vi "FrontPanel.vi"() -> ()   [LabVIEW 2016]
doc: "This VI controls the blindpanel type GHS-2T-1T-700 for a CryoFree DR. Automatization control is embedded in the blindpanel. Keys can be manipulated from within this VI."
uses:
  <userlib>/LevyLab/Leiden Tools/Leiden to DSC/FP to DSC/Typedefs/FP-cluster.ctl
  <vilib>/Utility/file.llb/Write Delimited Spreadsheet (string).vi
  Lib/Lib.llb/ErrCodeStatusLkup.vi
  Lib/Lib.llb/Pfeiffer Vacuum.lvlib
panel:
  out "VIRef":T1 {"Array DataType" format="%.0x"; "WaveForm Type" format="%.0x"; "RefNum Type" format="%.0x"; "DataType" format="%.0x"}
  out "ControlNames":string[](array[string])
  in  "Toolbar":enum32{"Page 1", "Page 2"}(tab)
  in  "Load config":bool
  in  "Save config":bool
  in  "Start":bool
  in  "Stop":bool
  out "V":string
  out "PT2 Data":dbl[](array[numeric])
  in  "Restart PT on Error?":bool
  in  "Attempts":u16=6
  in  "Time delay":u16=60 format="%.0f s"
  out "Error Log":string[][](table)
  in  "Error panel":enum32{"Page 1"}(tab)
  out "PT2 error":errorcluster
  out "MG error":errorcluster
  out "PT1 error":errorcluster
  out "FP error":errorcluster
  out "PT1 Data":dbl[](array[numeric])
  in  "Main Panel":enum32{"Page 1", "Page 2"}(tab)
  out "PC":sgl
  out "P1":sgl format="%.1f"
  out "P2":sgl format="%.1f"
  out "P3":sgl format="%.1f"
  out "P4":sgl format="%.1f"
  out "P5":sgl format="%.1f"
  out "P6":sgl format="%.1f"
  out "P7":sgl format="%.1f"
  out "Flow":sgl format="%#_4f"
  out "P5 alarm":bool
  out "Pstill (P8)":dbl format="%.1e"
  in  "Main Panel":T2(tab)
  out "String 2":string
  out "String 4":string
  out "String":string
  out "String 3":string
  out "Mode":u16(ring) items=["AUTO MODE OFF", "START", "CONDENSING 3He", "CONDENSING 4He", "NORMAL CIRCULATION", "RECOVERY OF THE MIXTURE", "RECOVERY: BLOCKAGE OR OVERPRESSURE"]
  out "FLOW":sgl format="%#_3f"
  out "P5":sgl
  out "P4":sgl
  out "P3":sgl
  out "P1":sgl
  out "P2":sgl
  out "3He":sgl(slide) min=0 max=2 scale=0.0..2000.0 scale format="%.2f"
  out "4He":sgl(slide) min=0 max=2 scale=0.0..2000.0 scale format="%.2f"
  out "Panel ID":string
  in  "FP type":enum32{"OLD", "NEW"}(tab)
  in  "Buttons":T3
  out "LEDs":T4
  in  "Buttons 2":T3
  out "LEDs 2":T5
  out "PC":sgl caption="P COMP"
  in  "PT Start 2":bool
  in  "PT_stop 2":bool
  in  "PT2 Plots Select":T6
  out "PT2 Status":cluster{"Time":dbl[], "Value":dbl[]}[](graph)
  in  "PT_ResetValues 2":bool
  out "PT Error Code 2":i32 caption="PT Error Code"
  out "PT Error 2":string="NO ERROR" caption="PT Error"
  out "P High":cluster{dbl, dbl, dbl, dbl}(slide) scale=150.0..450.0
  out "P Low":cluster{dbl, dbl, dbl, dbl}(slide) scale=0.0..300.0
  out "P_avg 2":cluster{"Low":dbl, "High":dbl} caption="Average pressure"
  out "Helium":cluster{dbl, dbl, dbl, dbl}(slide) scale=0.0..95.0
  out "Water In":cluster{dbl, dbl, dbl, dbl}(slide) scale=0.0..35.0
  out "Water Out":cluster{dbl, dbl, dbl, dbl}(slide) scale=0.0..60.0
  out "PT Status":u16(ring) items=["Compressor OFF", "Compressor ON", ""]
  out "Motor":cluster{dbl, dbl}(slide) scale=0.0..30.0
  out "Oil":cluster{dbl, dbl, dbl, dbl}(slide) scale=0.0..60.0
  in  "PT1 Plots Select":T6
  out "PT1 Status 2":cluster{"Time":dbl[], "Value":dbl[]}[](graph)
  out "P Low":cluster{dbl, dbl, dbl, dbl}(slide) scale=0.0..300.0
  out "P High":cluster{dbl, dbl, dbl, dbl}(slide) scale=150.0..450.0
  out "P_avg":cluster{"Low":dbl, "High":dbl} caption="Average pressure"
  out "Motor":cluster{dbl, dbl}(slide) scale=0.0..30.0
  out "Oil":cluster{dbl, dbl, dbl, dbl}(slide) scale=0.0..60.0
  out "Helium":cluster{dbl, dbl, dbl, dbl}(slide) scale=0.0..95.0
  out "Water Out":cluster{dbl, dbl, dbl, dbl}(slide) scale=0.0..60.0
  out "Water In":cluster{dbl, dbl, dbl, dbl}(slide) scale=0.0..35.0
  out "PT Error Code":i32
  out "PT Error":string="NO ERROR"
  in  "PT_ResetValues":bool
  in  "PT Start":bool
  in  "PT_stop":bool
  out "PT Status":u16(ring) items=["Compressor OFF", "Compressor ON", ""]
  in  "MG Plots Select":T6
  in  "FP Plots Select":T6
  out "MaxiGauge":cluster{"Time":dbl[], "Value":dbl[]}[](graph)
  out "Front Panel":cluster{"Time":dbl[], "Value":dbl[]}[](graph)
  in  "Boolean 2":bool
  out "Maxigauge ID":string
  out "ForceSave":bool
  in  "Type":enum32{"Wet", "CF"}(radio)=enum."CF"
  in  "Button":u8
  out "SetControl":T7
  in  "S2":enum32{"Page 1"}(tab)
  in  "Reset Error 2":bool
  in  "S1":enum32{"Page 1"}(tab)
  in  "Reset Error":bool
  out "Cur Path":path
  in  "Side Panel":enum32{"Main", "Settings", "Advanced"}(tab)=enum."Settings"
  out "Sensors Status":T8={"String 8"="OK", "String 9"="OK", "String 10"="OK", "String 11"="OK", "String 12"="OK", "String 13"="OK"}
  in  "ADC scaling":T9={"P1"=2500.0, "P2"=2500.0, "P3"=2500.0, "P4"=2500.0, "P5"=2500.0, "P6"=2500.0, "P7"=2500.0, "Flow meter"=682.0, "PC"=10000.0} caption="Front panel ADC scaling factors" {"Flow meter" format="%#.4f"}
  in  "REC Settings":T10={"P6 low"=20, "P6 high"=1000, "P7 low"=20}
  in  "NCP5B Settings":cluster{"P6 low":u16}={"P6 low"=20}
  in  "NCP5 Settings":T10={"P6 low"=20, "P6 high"=1000, "P7 low"=20}
  in  "S1&2 Settings":cluster{"Enum":enum16{"OFF", "ON"}}
  in  "P5 Settings":cluster{"P6 low":u16, "P6 high":u16}={"P6 low"=20, "P6 high"=1000}
  out "REC limits":T11={"P5 warn"=20, "P5 rec"=20, "P5 res"=20}
  out "NCP5B limits":cluster{"P5 NC4":u16}={"P5 NC4"=20}
  out "NCP5 limits":T12={"P5 NC1"=20, "P5 NC2"=20, "P5 NC3"=20}
  out "S1&2 limits":cluster{"S1&S2":enum16{"OFF", "ON"}}
  out "P5 limits":cluster{"P5 C1":u16, "P5 C2":u16}={"P5 C1"=20, "P5 C2"=20}
  in  "P6&7 Settings":T13={"P6 low"=20, "P6 high"=1600, "P7 low"=20, "P7 high"=1610}
  out "P6&7 limits":T13={"P6 low"=20, "P6 high"=20, "P7 low"=20, "P7 high"=20}
  in  "SET VALUES":bool
  out "MG pressures":T14 {"Channel 1" format="%-7.2e mbar"; "Channel 1" format="%-7.2e mbar"; "Channel 1" format="%-7.2e mbar"; "Channel 1" format="%-7.2e mbar"; "Channel 1" format="%-7.2e mbar"; "Channel 1" format="%-7.2e mbar"}
  out "Cluster":T15={"String 2"="\"\"", "String 3"="", "String 4"="", "String 5"="", "String 6"="", "String 7"=""}
  in  "Log Options":T16={"Plot data "=TRUE, "Every1"=1.0, "Save to log"=TRUE, "Every  2"=1.0, "AVS_Path 2"=path "C:/avs-47", "AVS_FName"="logFP", "Filename suffix"="_%Y-%m-%d-%H-%M-%S", "NewFevery"=7, "Time Units"=enum."Days", "Date Format"="%Y-%m-%d %H:%M:%S", "Averages"=4} caption="Data Logging \nOptions" {"Every  2" format="%#_g min"; "Every1" format="%#_g min"}
  in  "Configuration":T17={"FP port"="COM3", "MG port"="COM4", "PT1 Enabled?"=FALSE, "MG  channel P8"=65535, "Stop auto recovery if still is empty"=FALSE, "PT1 port"="COM2", "MG Enabled?"=TRUE, "PT1 Address"=16, "S1 Enabled?"=FALSE, "S1 port"="COM2", "S2 Enabled?"=FALSE, "S2 port"="COM2", "Device address S1"=1, "Device address S2"=2, "PT1 Bauds"=115200, "PT2 Enabled?"=FALSE, "PT2 port"="COM2", "PT2 Address"=16, "PT2 Bauds"=115200, "FP baud rate"=9600} {"PT2 Address" min=16 max=126 step=1; "MG  channel P8" items=["Channel 1", "Channel 2", "Channel 3", "Channel 4", "Channel 5", "Channel 6"]; "PT1 Address" min=16 max=126 step=1}
  in  "SendCMD":bool caption="Send"
  out "Response":string
  in  "Command":string
  out "SP reached? 2":bool
  in  "Cond1":bool
  in  "Delay Time":u32=30 caption="For a time delay of" format="%.0f min"
  in  "MG  channel":u16(ring)=65535 caption="MaxiGauge" items=["Channel 1", "Channel 2", "Channel 3", "Channel 4", "Channel 5", "Channel 6"]
  out "SP reached? 3":bool
  in  "P threshold":dbl=0.0005 caption="<" format="%#_2g mbar"
  in  "Cond2":bool
  out "SP reached?":bool
  out "Delay Timer":u32=10 caption="Timer" format="%<%M:%S>t"
  in  "EnableAutoCond":bool caption="Start"
  in  "Autoconf":bool caption="Autoconfigure"
  out "MG Data":dbl[](array[numeric]) format="%.3e"
  out "FP Data":sgl[](array[numeric]) format="%.2f"
  out "FP Status bits":u32[](array[numeric])
  out "Attempts Counter":u16
  # "Error log"
  # "Front panel status"
  # "MaxiGauge status"
  # "Pulse Tube 1 status"
  # "Pulse Tube 2 status"
  # "Leiden Cryogenics"
  # "to \nair"
  # "N.C."
  # "from\novc"
  # "from\nivc"
  # "from still"
  # "to 3He\nin-1"
  # "to 3He\nin-2"
  # "P8"
  # "AUX 1"
  # "MIXTURE\nCOMPRESSOR"
  # "M2"
  # "P6"
  # "M3"
  # "M1"
  # "AUX PORT-1"
  # "P7"
  # "TRAP"
  # "AUX TRAP"
  # "To \nAir"
  # "From\nIVC"
  # "From Still"
  # "To 3He\nin-1"
  # "To 3He\nin-2"
  # "To \nAir"
  # "N.C."
  # "from\novc"
  # "from\nivc"
  # "from still"
  # "to 3He\nin-1"
  # "to 3He\nin-2"
  # "Leiden Cryogenics"
  # "to \nair"
  # "N.C."
  # "from\novc"
  # "from\nivc"
  # "from still"
  # "to 3He\nin-1"
  # "to 3He\nin-2"
  # "P8"
  # "M2"
  # "P6"
  # "M3"
  # "TRAP"
  # "AUX TRAP"
  # "M1"
  # "AUX PORT-1"
  # "P7"
  # "AUX 1"
  # "To \nAir"
  # "From\nIVC"
  # "From Still"
  # "To 3He\nin-1"
  # "to 3He\nin-1"
  # "To 3He\nin-2"
  # "to \nair"
  # "N.C."
  # "from\novc"
  # "from\nivc"
  # "from still"
  # "to 3He\nin-2"
  # "Pulse Tube 1"
  # "Pulse Tube 2"
  # "Front Panel"
  # "MaxiGauge"
  # "Turbo2 (S2)"
  # "Turbo1 (S1)"
  # "MaxiGauge"
  # "#"
  # "NAME"
  # "PRESSURE"
  # "STATUS"
  # "1"
  # "2"
  # "3"
  # "4"
  # "5"
  # "6"
  # "Automatic mode pressure limits"
  # "Warning: These values influence the operation of the GHS in automatic mode. Please refer to the operation manual and consult with Leiden Cryogenics before changing them."
  # "NAME"
  # "FW"
  # "NEW"
  # "DESCRIPTION"
  # "Stop condensing 4He"
  # "Stop recovering 4He"
  # "Stop condensing 3He"
  # "Stop recovering 3He"
  # "Condensing->open 12"
  # "Condensing->close 9/12"
  # "Condensing->run S1&S2"
  # "NC->open second line"
  # "NC->start MC"
  # "NC->open aux. trap"
  # "NC->stop MC, close 7"
  # "All->P5 alarm"
  # "All->switch to recovery"
  # "All->reset"
  # "Front panel ADC scaling factors"
  # "Data Logging and Plotting"
  # "Front Panel"
  # "MaxiGauge"
  # "Pulse Tube 1"
  # "Pulse Tube 2"
  # "Turbo 1 (S1) (Pfeiffer HiPACE only)"
  # "Turbo2 (S2) (Pfeiffer HiPACE only)"
  # "Automatic condensing"
  # "Start condensing when"
  # "and wait"
  # "Send command to Front Panel"
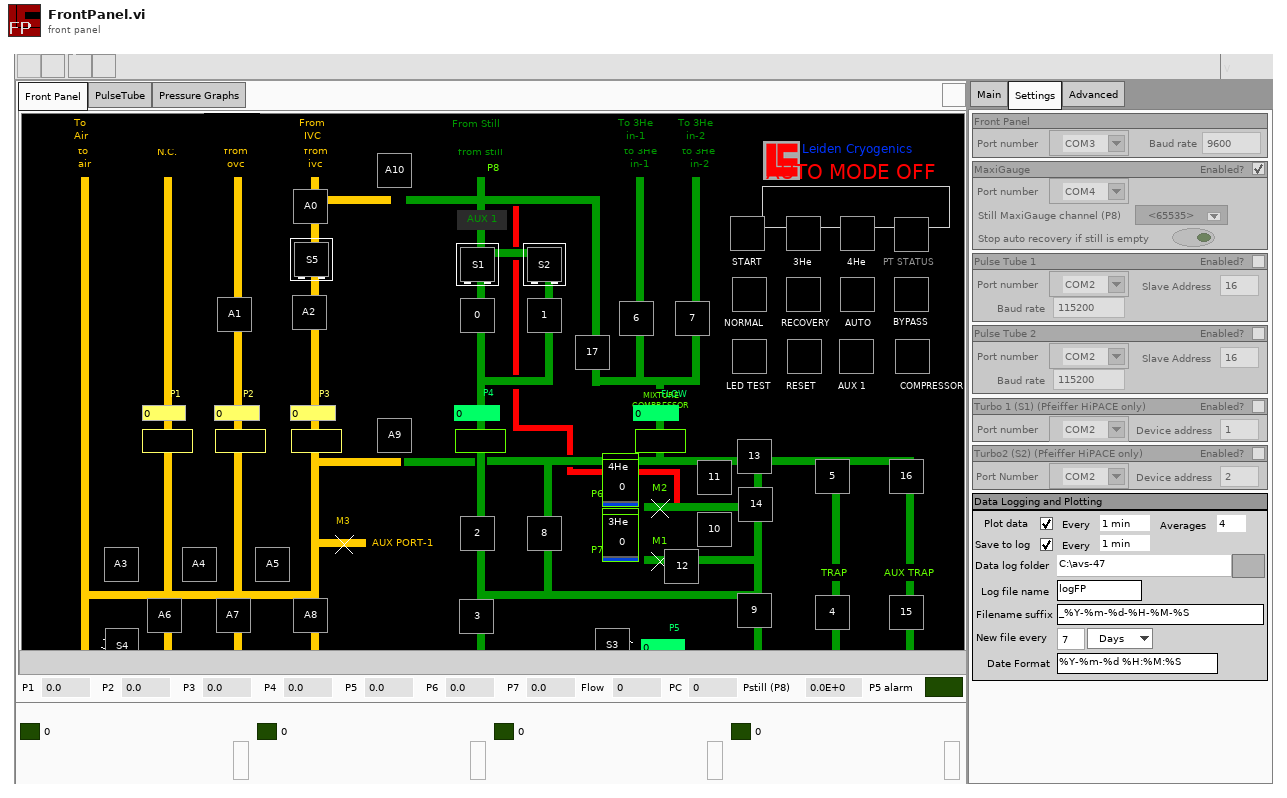
[diagram p1: front panel]
types:
  T1 = cluster{"Control Ref ID":refnum<vi>[], "Full Name":string[], "ClassID":enum16{"<Null>", "1", "2", "Generic", "Decoration", "Text", "Control", "ColorBox", "Boolean", "RefNum", "Variant", "Path", "ListBox", "Table", "Array", "Picture", "ActiveXContainer", "Numeric", "Digital", "NamedNumeric", "ColorRamp", "Slide", "GraphOrChart", "WaveformChart", "WaveformGraph", "IntensityChart", "IntensityGraph", "String", "IOName", "ComboBox", "Cluster", "Panel", "Knob", "NumWithScale", "Ring", "Enum", "GObject", "Plot", "Cursor", "NumericText", "Scale", "ColorScale", "GraphScale", "ColorGraphScale", "TypedRefNum", "OldKnobScale", "MCListbox", "MeasureData", "BVTag", "DAQName", "VISAName", "IVIName", "SlideScale", "TabControl", "Page", "TabArrayTabControl", "ConPane", "57", "58", "59", "60", "61", "62", "63", "64", "SubPanel", "TreeControl", "67", "68", "69", "70", "71", "72", "73", "74", "75", "SplitterBar"}[], "Short Name":string[], "DataType":enum8{"<Null>", "I8", "I16", "I32", "I64", "U8", "U16", "U32", "U64", "SGL", "DBL", "EXT", "CSG", "CDB", "CXT", "0x0F", "0x10", "0x11", "0x12", "0x13", "0x14", "Enum U8", "Enum U16", "Enum U32", "Enum U64", "SGL PQ", "DBL PQ", "EXT PQ", "CSG PQ", "CDB PQ", "CXT PQ", "0x1F", "0x20", "Boolean", "0x22", "0x23", "0x24", "0x25", "0x26", "0x27", "0x28", "0x29", "0x2A", "0x2B", "0x2C", "0x2D", "0x2E", "0x2F", "String", "0x31", "Path", "Pict", "0x34", "0x35", "0x36", "DAQ", "0x38", "0x39", "0x3A", "0x3B", "0x3C", "0x3D", "0x3E", "0x3F", "Array", "0x41", "0x42", "0x43", "0x44", "0x45", "0x46", "0x47", "0x48", "0x49", "0x4A", "0x4B", "0x4C", "0x4D", "0x4E", "0x4F", "Cluster", "0x51", "0x52", "Variant", "Waveform", "0x55", "0x56", "0x57", "0x58", "0x59", "0x5A", "0x5B", "0x5C", "0x5D", "0x5E", "0x5F", "0x60", "0x61", "0x62", "0x63", "0x64", "0x65", "0x66", "0x67", "0x68", "0x69", "0x6A", "0x6B", "0x6C", "0x6D", "0x6E", "0x6F", "Refnum"}[], "RefNum Type":enum8{"Generic", "Datalog File Refnum", "Byte Stream File Refnum", "Device Refnum", "Occurence Refnum", "TCP Connection Refnum", "VISA Refnum (Obsolete)", "Automation Renum", "VI Server Refnum", "Menu Refnum", "IVI Refnum (Obsolete)", "IMAQ Session", "0x0C", "Datasocket Refnum", "VISA Resource", "IVI Logical Name", "UDP Connection Refnum", "Notifier Refnum", "Queue Refnum", "IrDA Refnum", "Hardware Plugin Refnum", "Hardware Plugin Tag Refnum", "DAQmx Refnum", "Event Registration Refnum", ".NET Refnum", "User Event Refnum", "0x1A", "Event Callback", "0x1C", "0x1D", "Only Used Internal to LabVIEW", "Bluetooth", "Data Value References", "RT FIFO", "TDM Streaming"}[], "WaveForm Type":enum8{"<Not a Waveform Type>", "0x01", "Analog 16-bit signed", "Analog Double-Precision", "0x04", "Analog Single Precision", "Timestamp", "Digital Data", "Digital Waveform", "Dynamic Data", "Analog Extended-Precision", "Analog 8-bit unsigned", "Analog 16-bit unsigned", "Analog 32-bit unsigned", "Analog 8-bit signed", "Analog 32-bit signed", "Analog Complex Single-Precision", "Analog Complex Double-Precision", "Analog Complex Extended Precision", "Analog 64-bit signed", "Analog 64-bit unsigned"}[], "Parent":i32[], "Array DataType":enum8{"<Null>", "I8", "I16", "I32", "I64", "U8", "U16", "U32", "U64", "SGL", "DBL", "EXT", "CSG", "CDB", "CXT", "0x0F", "0x10", "0x11", "0x12", "0x13", "0x14", "Enum U8", "Enum U16", "Enum U32", "Enum U64", "SGL PQ", "DBL PQ", "EXT PQ", "CSG PQ", "CDB PQ", "CXT PQ", "0x1F", "0x20", "Boolean", "0x22", "0x23", "0x24", "0x25", "0x26", "0x27", "0x28", "0x29", "0x2A", "0x2B", "0x2C", "0x2D", "0x2E", "0x2F", "String", "0x31", "Path", "Pict", "0x34", "0x35", "0x36", "DAQ", "0x38", "0x39", "0x3A", "0x3B", "0x3C", "0x3D", "0x3E", "0x3F", "Array", "0x41", "0x42", "0x43", "0x44", "0x45", "0x46", "0x47", "0x48", "0x49", "0x4A", "0x4B", "0x4C", "0x4D", "0x4E", "0x4F", "Cluster", "0x51", "0x52", "Variant", "Waveform", "0x55", "0x56", "0x57", "0x58", "0x59", "0x5A", "0x5B", "0x5C", "0x5D", "0x5E", "0x5F", "0x60", "0x61", "0x62", "0x63", "0x64", "0x65", "0x66", "0x67", "0x68", "0x69", "0x6A", "0x6B", "0x6C", "0x6D", "0x6E", "0x6F", "Refnum"}[], "Owning VI":refnum<vi>[], "Active?":bool[]}
  T2 = enum32{"Front Panel", "PulseTube", "Pressure Graphs"}
  T3 = cluster{"baux2":bool, "bBypass":bool, "b15":bool, "b16":bool, "NC 0":bool, "baux1":bool, "b4":bool, "NC 1":bool, "b5":bool, "breset":bool, "NC 2":bool, "b9":bool, "b14":bool, "NC 3":bool, "b13":bool, "bledtest":bool, "NC 4":bool, "b12":bool, "b10":bool, "NC 5":bool, "b11":bool, "bA0":bool, "NC 9":bool, "b7":bool, "bS3":bool, "NC 12":bool, "b6":bool, "b17":bool, "NC 13":bool, "b8":bool, "b1":bool, "NC 14":bool, "bS2":bool, "b3":bool, "NC 15":bool, "b2":bool, "b0":bool, "NC 16":bool, "bS1":bool, "bA9":bool, "NC 17":bool, "bA8":bool, "bA2":bool, "NC 6":bool, "bs5":bool, "bA10":bool, "NC 7":bool, "bstart":bool, "bA5":bool, "NC 8":bool, "bA7":bool, "bA1":bool, "NC 10":bool, "bauto":bool, "bA4":bool, "NC 11":bool, "bA6":bool, "bS4":bool, "NC 18":bool, "bA3":bool, "b3he":bool, "b4he":bool, "bnorm":bool, "brecov":bool}
  T4 = cluster{"COMPR/AUX 2":bool, "BYPASS":bool, "15":bool, "16":bool, "NC 0":bool, "AUX 1":bool, "4":bool, "NC 1":bool, "5":bool, "RESET":bool, "NC 2":bool, "9":bool, "14":bool, "NC 3":bool, "13":bool, "LED TEST":bool, "NC 4":bool, "12":bool, "10":bool, "NC 5":bool, "11":bool, "A0":bool, "NC 12":bool, "7":bool, "S3":bool, "NC 13":bool, "6":bool, "17":bool, "NC 14":bool, "8":bool, "1":bool, "NC 15":bool, "S2":bool, "3":bool, "NC 16":bool, "2":bool, "0":bool, "NC 17":bool, "S1":bool, "A9":bool, "NC 6":bool, "A8":bool, "A2":bool, "NC 7":bool, "S5":bool, "A10":bool, "NC 8":bool, "START":bool, "A5":bool, "NC 9":bool, "A7":bool, "A1":bool, "NC 10":bool, "AUTO":bool, "A4":bool, "NC 11":bool, "A6":bool, "S4":bool, "NC 18":bool, "A3":bool, "3He":bool, "4He":bool, "NORMAL":bool, "RECOVERY":bool, "PT STATUS":bool}
  T5 = cluster{"COMPR/AUX 2":bool, "BYPASS":bool, "15":bool, "16":bool, "AUX 1":bool, "AUX 1":bool, "4":bool, "AUX 2":bool, "5":bool, "RESET":bool, "AUX 3":bool, "9":bool, "14":bool, "NC 3":bool, "13":bool, "LED TEST":bool, "NC 4":bool, "12":bool, "10":bool, "NC 5":bool, "11":bool, "A0":bool, "NC 12":bool, "7":bool, "S3":bool, "NC 13":bool, "6":bool, "17":bool, "NC 14":bool, "8":bool, "1":bool, "NC 15":bool, "S2":bool, "3":bool, "NC 16":bool, "2":bool, "0":bool, "NC 17":bool, "S1":bool, "A9":bool, "NC 6":bool, "A8":bool, "A2":bool, "NC 7":bool, "S5":bool, "A10":bool, "NC 8":bool, "START":bool, "A5":bool, "NC 9":bool, "A7":bool, "A1":bool, "NC 10":bool, "AUTO":bool, "A4":bool, "NC 11":bool, "A6":bool, "S4":bool, "NC 18":bool, "A3":bool, "3He":bool, "4He":bool, "NORMAL":bool, "RECOVERY":bool, "PT STATUS":bool}
  T6 = cluster{"Boolean":bool, "Boolean 2":bool, "Boolean 3":bool, "Boolean 4":bool, "Boolean 5":bool, "Boolean 6":bool, "Boolean 7":bool, "Boolean 8":bool}
  T7 = cluster{"Name":string, "Scalar":string, "Array":string[][]}
  T8 = cluster{"String 8":string, "String 9":string, "String 10":string, "String 11":string, "String 12":string, "String 13":string}
  T9 = cluster{"P1":dbl, "P2":dbl, "P3":dbl, "P4":dbl, "P5":dbl, "P6":dbl, "P7":dbl, "Flow meter":dbl, "PC":dbl}
  T10 = cluster{"P6 low":u16, "P6 high":u16, "P7 low":u16}
  T11 = cluster{"P5 warn":u16, "P5 rec":u16, "P5 res":u16}
  T12 = cluster{"P5 NC1":u16, "P5 NC2":u16, "P5 NC3":u16}
  T13 = cluster{"P6 low":u16, "P6 high":u16, "P7 low":u16, "P7 high":u16}
  T14 = cluster{"Channel 1":dbl, "Channel 1":dbl, "Channel 1":dbl, "Channel 1":dbl, "Channel 1":dbl, "Channel 1":dbl}
  T15 = cluster{"String 2":string, "String 3":string, "String 4":string, "String 5":string, "String 6":string, "String 7":string}
  T16 = cluster{"Plot data ":bool, "Every1":dbl, "Save to log":bool, "Every  2":dbl, "AVS_Path 2":path, "AVS_FName":string, "Filename suffix":string, "NewFevery":u32, "Time Units":enum16{"Minutes", "Hours", "Days"}, "Date Format":string, "Averages":i32}
  T17 = cluster{"FP port":refnum<visa-resource-name>, "MG port":refnum<visa-resource-name>, "PT1 Enabled?":bool, "MG  channel P8":u16, "Stop auto recovery if still is empty":bool, "PT1 port":refnum<visa-resource-name>, "MG Enabled?":bool, "PT1 Address":u8, "S1 Enabled?":bool, "S1 port":refnum<visa-resource-name>, "S2 Enabled?":bool, "S2 port":refnum<visa-resource-name>, "Device address S1":u8, "Device address S2":u8, "PT1 Bauds":u32, "PT2 Enabled?":bool, "PT2 port":refnum<visa-resource-name>, "PT2 Address":u8, "PT2 Bauds":u32, "FP baud rate":u32}
  T18 = typedef "FP-cluster.ctl" = cluster{"FP Data":sgl[], "MG Data":dbl[], "PT Data":dbl[], "FP Status Bits":u32[], "Mode":u16}
  T19 = cluster{"error":bool, "code":i32, "source":string}
  T20 = cluster{"FP Data[0]":sgl, "FP Data[1]":sgl, "FP Data[2]":sgl, "FP Data[3]":sgl, "FP Data[4]":sgl, "FP Data[5]":sgl, "FP Data[6]":sgl, "FP Data[7]":sgl, "FP Data[8]":sgl}
  T21 = enum32{"Page Enabled", "Page Disabled", "Page Disabled & Grayed"}
  T22 = enum32{"invalid app kind", "Development System", "Run Time System", "Student Edition", "Embedded LabVIEW", "Evaluation", "Custom"}
  T23 = enum32{"HKEY_CLASSES_ROOT", "HKEY_CURRENT_USER", "HKEY_LOCAL_MACHINE", "HKEY_USERS", "HKEY_PERFORMANCE_DATA", "HKEY_CURRENT_CONFIG", "HKEY_DYN_DATA"}
  T24 = cluster{"Array[0]":string, "Array[1]":string, "Array[2]":string, "Array[3]":string, "Array[4]":string, "Array[5]":string}
  T25 = cluster{"array of 4 x 16 bit unsigned[0]":u16, "array of 4 x 16 bit unsigned[1]":u16, "array of 4 x 16 bit unsigned[2]":u16, "array of 4 x 16 bit unsigned[3]":u16}
  T26 = cluster{"array of 2 x 16 bit unsigned[0]":u16, "array of 2 x 16 bit unsigned[1]":u16}
  T27 = cluster{"array of 3 x 16 bit unsigned[0]":u16, "array of 3 x 16 bit unsigned[1]":u16, "array of 3 x 16 bit unsigned[2]":u16}
  T28 = typedef "LVRectTypeDef.ctl" = cluster{"Left":i16, "Top":i16, "Right":i16, "Bottom":i16}
  T29 = cluster{"[0]":bool, "[1]":bool, "[2]":bool, "[3]":bool, "[4]":bool, "[5]":bool, "[6]":bool, "[7]":bool, "[8]":bool, "[9]":bool, "[10]":bool, "[11]":bool, "[12]":bool, "[13]":bool, "[14]":bool, "[15]":bool, "[16]":bool, "[17]":bool, "[18]":bool, "[19]":bool, "[20]":bool, "[21]":bool, "[22]":bool, "[23]":bool, "[24]":bool, "[25]":bool, "[26]":bool, "[27]":bool, "[28]":bool, "[29]":bool, "[30]":bool, "[31]":bool, "[32]":bool, "[33]":bool, "[34]":bool, "[35]":bool, "[36]":bool, "[37]":bool, "[38]":bool, "[39]":bool, "[40]":bool, "[41]":bool, "[42]":bool, "[43]":bool, "[44]":bool, "[45]":bool, "[46]":bool, "[47]":bool, "[48]":bool, "[49]":bool, "[50]":bool, "[51]":bool, "[52]":bool, "[53]":bool, "[54]":bool, "[55]":bool, "[56]":bool, "[57]":bool, "[58]":bool, "[59]":bool, "[60]":bool, "[61]":bool, "[62]":bool, "[63]":bool, "[64]":bool}
  T30 = cluster{"Dict. Var":u16, "Description":string, "Values":i32[]}[]
  T31 = cluster{"[3]":dbl, "[3]":dbl, "[3]":dbl, "Values[3] 2":dbl}
  T32 = cluster{"[1]":dbl, "[1]":dbl, "[1]":dbl, "Values[1] 2":dbl}
  T33 = cluster{"Values[0]":dbl, "Values[0]":dbl, "Values[0]":dbl, "Values[0] 2":dbl}
  T34 = cluster{"error":bool, "code":i32, "error source":string}
  T35 = cluster{"sensor status info[0]":string, "sensor status info[1]":string, "sensor status info[2]":string, "sensor status info[3]":string, "sensor status info[4]":string, "sensor status info[5]":string}
  T36 = cluster{"Filterred[0]":dbl, "Filterred[1]":dbl, "Filterred[2]":dbl, "Filterred[3]":dbl, "Filterred[4]":dbl, "Filterred[5]":dbl}
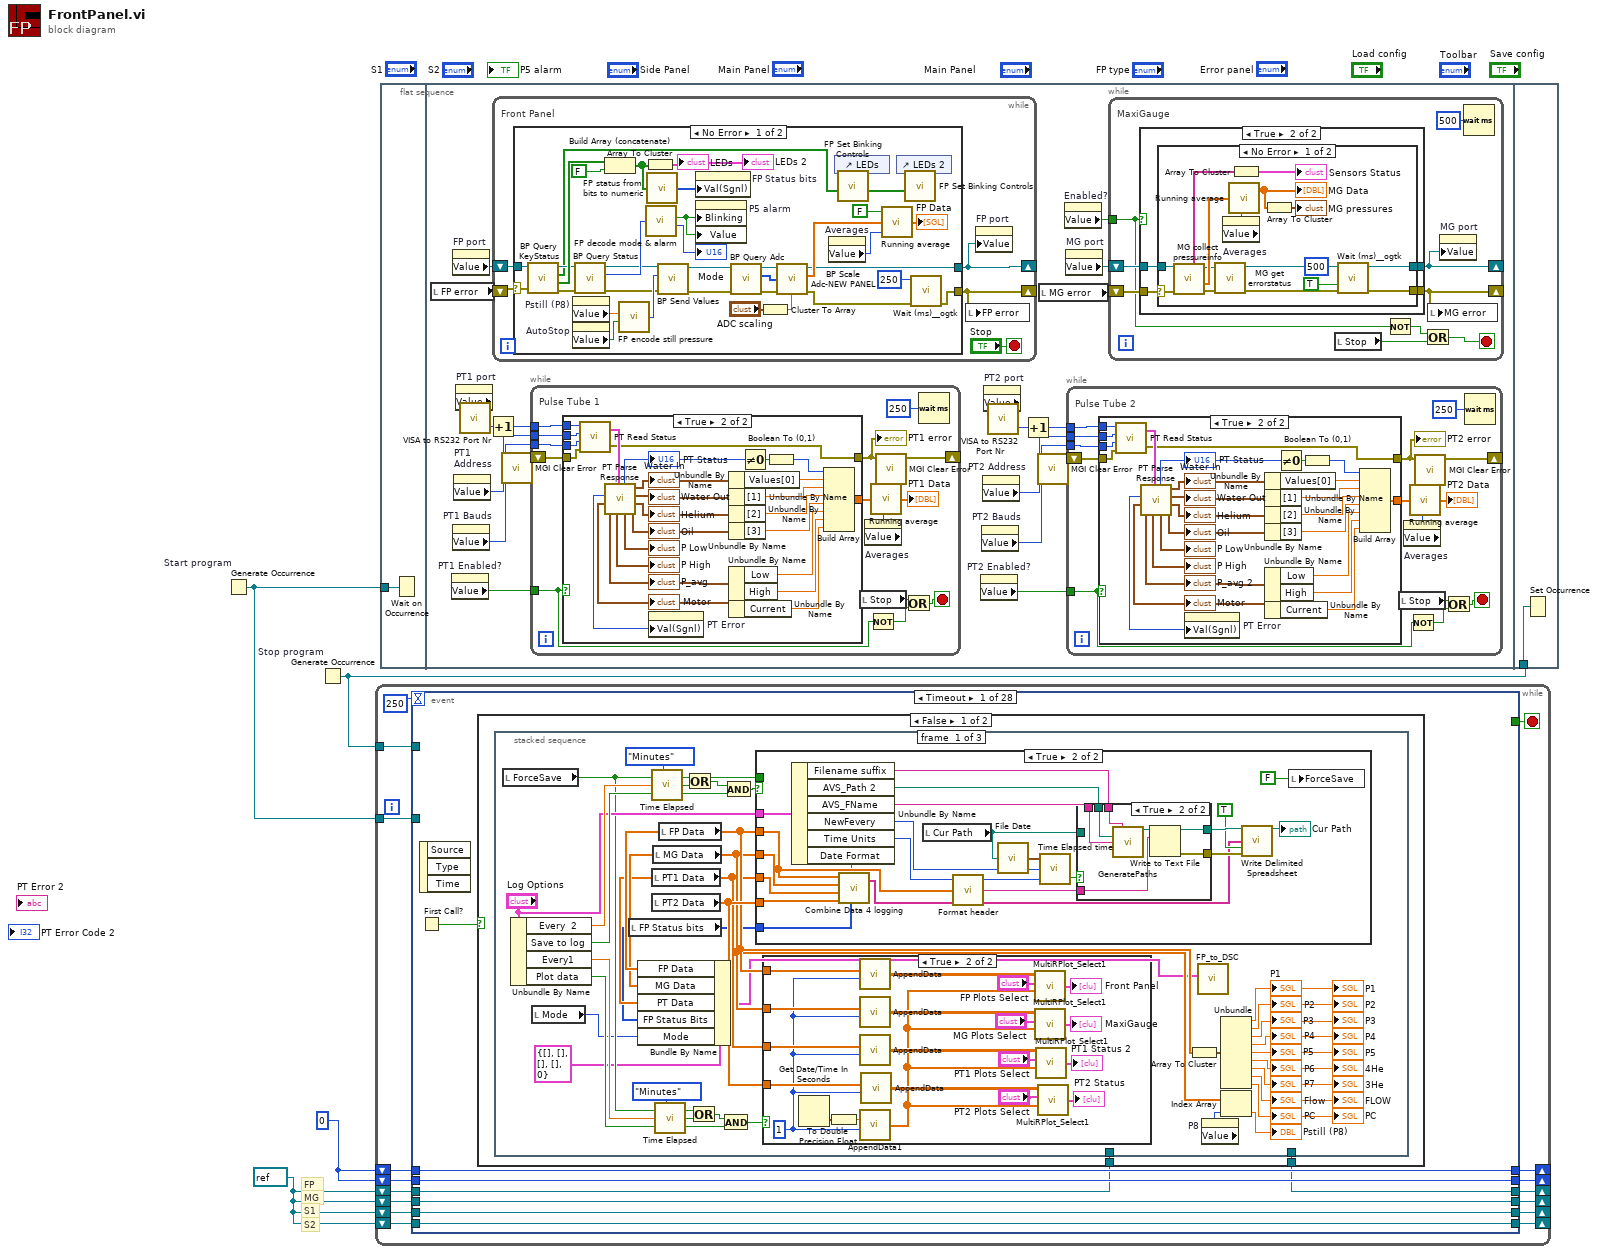
[diagram p0: block diagram]
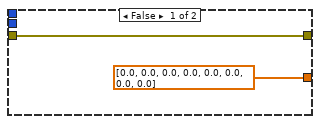
[diagram p2: hidden frame]
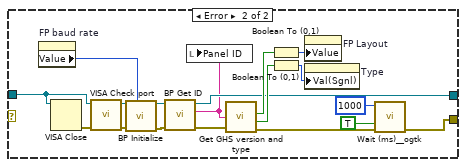
[diagram p3: hidden frame]
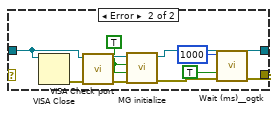
[diagram p5: hidden frame]
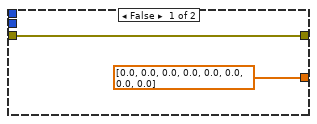
[diagram p6: hidden frame]
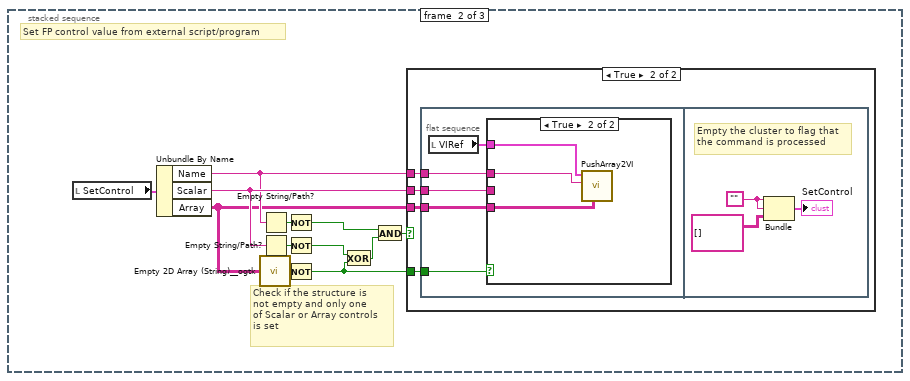
[diagram p10: hidden frame]
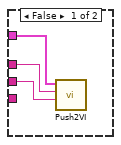
[diagram p12: hidden frame]
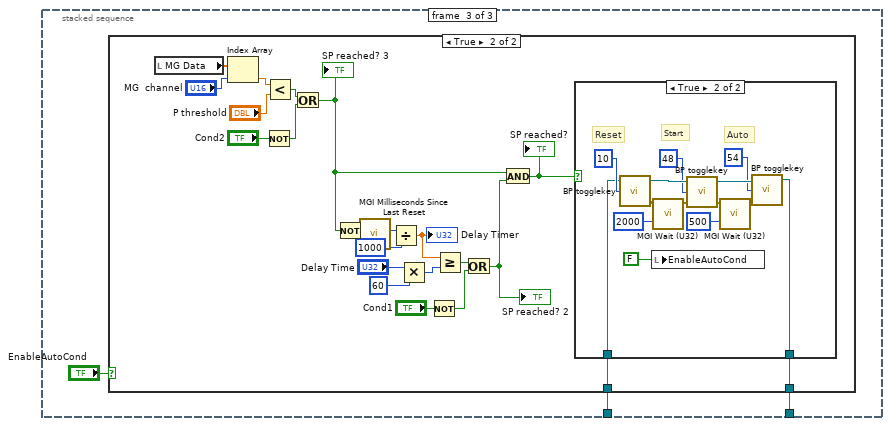
[diagram p13: hidden frame]
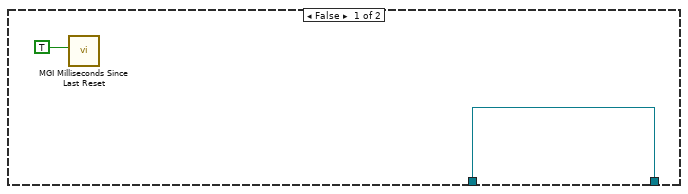
[diagram p14: hidden frame]
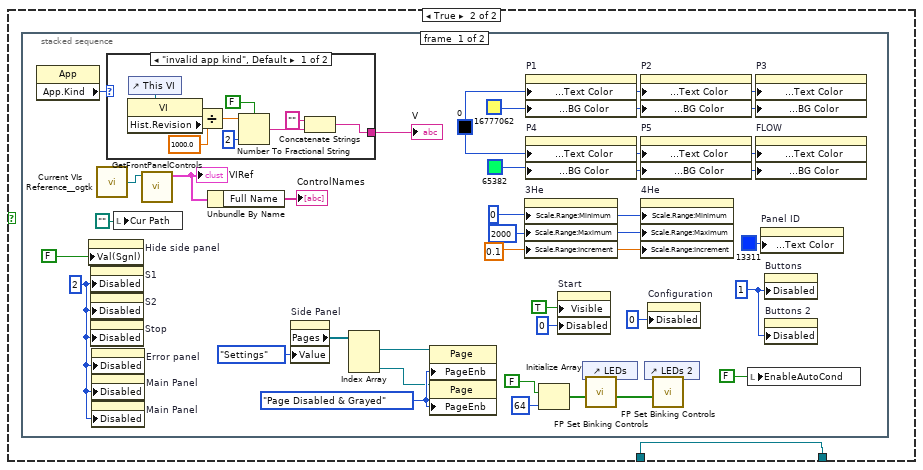
[diagram p16: hidden frame]
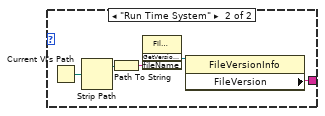
[diagram p17: hidden frame]
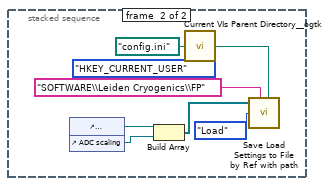
[diagram p18: hidden frame]
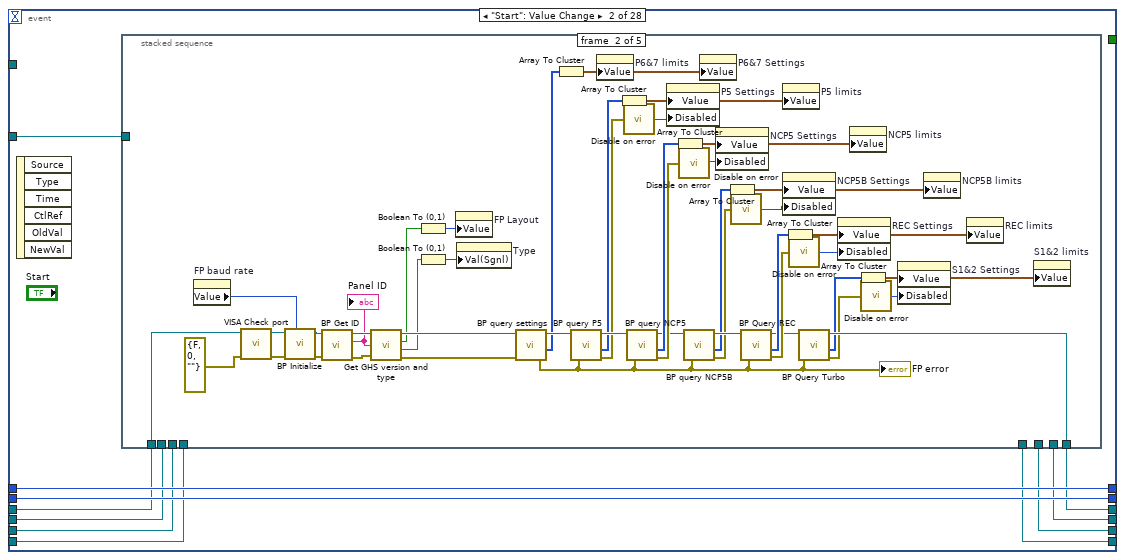
[diagram p19: hidden frame]
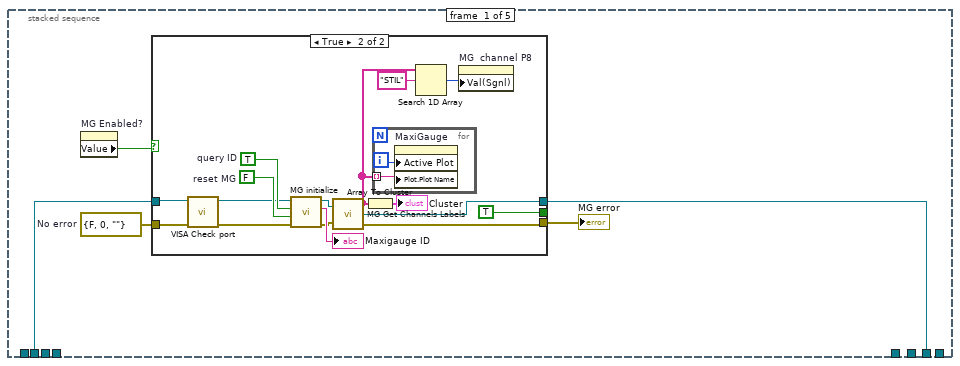
[diagram p20: hidden frame]
diagram:
  w3 = refnum<visa-resource-name> refnum ("PT port")
  w1 = u8 0
  # "S2"
  # "S1"
  # "FP"
  # "MG"
  n1 = Generate Occurrence "Start program"() -> (w4:refnum<k4>)
  n2 = Generate Occurrence "Stop program"() -> (w2:refnum<k4>)
  n3 = while {
    shift-right: [w12] -> _
    shift-left: w3 -> [w18]
    shift-right: [w16] -> _
    shift-left: w3 -> [w17]
    tunnel: w4 -> [w15]
    shift-right: [w13] -> _
    shift-left: w1 -> [w14]
    shift-right: [w9] -> _
    shift-left: w3 -> [w11]
    shift-right: [w8] -> _
    shift-left: w3 -> [w10]
    tunnel: w2 -> [w7]
    shift-right: [w5] -> _
    shift-left: w1 -> [w6]
    stop <- w20 stop-if-true
    n4 = event shown="[0] Timeout" {
      selector: _ -> [_ _ _ _ _ _ _ _ _ _ _ _ _ _ _ _ _ _ _ _ _ _ _ _ _ _ _ _]
      dyn-events: _ -> [_ _ _ _ _ _ _ _ _ _ _ _ _ _ _ _ _ _ _ _ _ _ _ _ _ _ _ _]
      timeout: 250 -> [_ _ _ _ _ _ _ _ _ _ _ _ _ _ _ _ _ _ _ _ _ _ _ _ _ _ _ _]
      tunnel: [_ _ TRUE _ _ _ _ _ _ _ _ _ _ _ _ _ _ _ _ _ _ _ _ _ _ _ _ _] -> w20
      tunnel: w18 -> [w22 w244 w349 w373 w382 w391 w400 w412 w443 w452 w458 w471 w485 w489 w582 w591 w601 w620 w634 w654 w664 w679 w686 w694 w702 w713 w725 w746]
      tunnel: w17 -> [w24 w246 w348 w372 w381 w390 w399 w411 w442 w451 w456 w469 w483 w493 w581 w590 w602 w619 w633 w653 w663 w678 w687 w695 w701 w712 w723 w749]
      tunnel: [w24 w245 w343 w372 w381 w390 w399 w411 w442 w451 w456 w469 w483 w493 w581 w590 w600 w619 w633 w653 w663 w678 w687 w695 w701 w712 w723 w749] -> w16
      tunnel: w15 -> [_ w242 _ _ _ _ _ _ _ _ _ _ _ _ _ _ _ _ _ _ _ _ _ _ _ _ _ _]
      tunnel: w14 -> [w27 w247 _ w371 w380 w389 w398 w408 w441 w450 w464 w476 w487 w492 w580 w592 _ w621 w635 w652 w665 w675 w685 w693 w703 w714 w724 w751]
      tunnel: [w27 w247 w344 w371 w380 w389 w398 w408 w441 w450 w464 w476 w487 w492 w580 w592 w603 w621 w635 w652 w665 w675 w685 w693 w703 w714 w724 w751] -> w13
      tunnel: [w21 w243 w343 w373 w382 w391 w400 w412 w443 w452 w457 w470 w484 w488 w582 w591 w606 w620 w634 w654 w664 w679 w686 w694 w702 w713 w725 w745] -> w12
      tunnel: w11 -> [w26 w241 w347 w370 w379 w388 w397 w404 w440 w449 w455 w468 w482 w491 w579 w589 w599 w618 w632 w651 w662 w677 w689 w696 w700 w711 w722 w748]
      tunnel: w10 -> [w25 w240 w346 w369 w378 w387 w396 w403 w439 w448 w454 w467 w481 w490 w578 w588 w597 w617 w631 w650 w661 w676 w688 w697 w699 w710 w721 w747]
      tunnel: [w26 w239 w343 w370 w379 w388 w397 w404 w440 w449 w455 w468 w482 w491 w579 w589 w598 w618 w632 w651 w662 w677 w683 w696 w700 w711 w722 w748] -> w9
      tunnel: [w25 w238 w343 w369 w378 w387 w396 w403 w439 w448 w454 w467 w481 w490 w578 w588 w596 w617 w631 w650 w661 w676 w688 w691 w699 w710 w721 w747] -> w8
      tunnel: w7 -> [_ _ w345 _ _ _ _ _ _ _ _ _ _ _ _ _ _ _ _ _ _ _ _ _ _ _ _ _]
      tunnel: w6 -> [w23 w248 _ w368 w377 w386 w395 w402 w438 w447 w463 w477 w486 w495 w577 w587 _ w608 w630 w640 w657 w674 w682 w690 w698 w709 w720 w750]
      tunnel: [w23 w248 w344 w368 w377 w386 w395 w402 w438 w447 w463 w477 w486 w495 w577 w587 w594 w608 w630 w640 w657 w674 w682 w690 w698 w709 w720 w750] -> w5
      event Timeout {
        n5 = First Call?() -> (First Call?: T/F=w28:bool)
        n6 = event-data() -> ()  [unwired: 1 in, 3 out]
        n7 = case shown="False" w28 {
          tunnel: w22 -> [w30 w186]
          tunnel: [w29 w186] -> w21
          frame False {
            n8 = stacked-sequence {
              tunnel: w30 -> [_ _ w145]
              tunnel: [_ _ w144] -> w29
              frame #0 {
                n9 = local read "ForceSave"() -> (w42:bool)
                n10 = Unbundle By Name("Log Options") -> ("Every  2"=w50:dbl, "Save to log"=w51:bool, "Every1"=w41:dbl, "Plot data"=w52:bool)
                n11 = local read "Mode"() -> (w32:u16)
                n12 = local read "FP Status bits"() -> (w33:u32[])
                n13 = call "Time Elapsed.vi"("Every"=w50, "Time Units"=enum16{"Minutes", "Hours", "Days"}."Minutes") -> ("Triggered?"=w46:bool)  [unwired: 1 in]
                n14 = local read "PT1 Data"() -> (w34:dbl[])
                n15 = local read "PT2 Data"() -> (w40:dbl[])
                n16 = local read "MG Data"() -> (w35:dbl[])
                n17 = call "Time Elapsed.vi"("Every"=w41, "Time Units"=enum16{"Minutes", "Hours", "Days"}."Minutes") -> ("Triggered?"=w45:bool)  [unwired: 1 in]
                n18 = local read "FP Data"() -> (w36:sgl[])
                n19 = Bundle By Name(cluster=T18 {"FP Data"=[], "MG Data"=[], "PT Data"=[], "FP Status Bits"=[], "Mode"=0} ("FP cluster"), "FP Data"=w36, "MG Data"=w35, "PT Data"=w34, "FP Status Bits"=w33, "Mode"=w32) -> (w31:T18)
                n20 = Or(x=w42, y=w46) -> (x .or. y?=w44:bool)
                n21 = Or(x=w42, y=w45) -> (x .or. y?=w43:bool)
                n22 = And(x=w43, y=w52) -> (x .and. y?=w63:bool)
                n23 = And(x=w44, y=w51) -> (x .and. y?=w64:bool)
                n24 = case shown="True" w64 {
                  tunnel: w36 -> [_ w93]
                  tunnel: w35 -> [_ w105]
                  tunnel: w33 -> [_ w104]
                  tunnel: w34 -> [_ w106]
                  tunnel: "Log Options" -> [_ w99]
                  tunnel: w42 -> [_ _]
                  tunnel: w40 -> [_ w87]
                  frame False {
                  }
                  frame True {
                    n25 = Unbundle By Name(w99) -> ("Filename suffix"=w96:string, "AVS_Path 2"=w98:path, "AVS_FName"=w97:string, "NewFevery"=w91:u32, "Time Units"=w90:enum16{"Minutes", "Hours", "Days"}, "Date Format"=w89:string)
                    n26 = call "Combine Data 4 logging.vi"("FP Status Bits"=w104, "Time Format String"=w89, "PT2 Data"=w87, "PT1 Data"=w106, "MG Data"=w105, "FP Data"=w93) -> ("Array"=w85:string[])  [unwired: 1 in]
                    n27 = local read "Cur Path"() -> (w94:path)
                    n28 = call "Format header.vi"("FP Data"=w93) -> ("Header string"=w92:string)  [unwired: 4 in]
                    n29 = call "File Date.vi"("Cur Path"=w94) -> ("Time Stamp"=w103:timestamp)  [unwired: 4 in]
                    n30 = call "Time Elapsed time.vi"("Time Units"=w90, "Delay Time"=w91, "Time Old In"=w103) -> ("T>dT?"=w95:bool)  [unwired: 2 out]
                    n31 = case shown="True" w95 {
                      tunnel: [w107 w109] -> w101
                      tunnel: [_ w113] -> w100
                      tunnel: w98 -> [_ w112]
                      tunnel: w97 -> [_ w111]
                      tunnel: w96 -> [_ w110]
                      tunnel: w94 -> [w107 _]
                      tunnel: w92 -> [_ w108]
                      frame False {
                      }
                      frame True {
                        n32 = call "GeneratePaths.vi"("Filename Suffix"=w110, "AVS_Path"=w112, "AVS_FName"=w111) -> ("Generated Log path"=w109:path)  [unwired: 11 in, 1 out]
                        n33 = Write to Text File(file (use dialog)=w109, text=w108) -> (error out=w113:errorcluster)  [unwired: 2 in, 2 out]
                      }
                    }
                    n34 = call-poly <vilib>:"Write Delimited Spreadsheet.vi"("file path (dialog if empty)"=w101, "1D data"=w85, "append to file? (new file:F)"=TRUE, "error in (no error)"=w100) -> ("new file path (Not A Path if cancelled)"=→"Cur Path":path)  [unwired: 10 in, 1 out]
                    n35 = local write "ForceSave"(FALSE ("ForceSave")) -> ()
                  }
                }
                n36 = case shown="True" w63 {
                  tunnel: w35 -> [_ w74]
                  tunnel: w36 -> [_ w84]
                  tunnel: w34 -> [_ w75]
                  tunnel: w40 -> [_ w68]
                  frame False {
                  }
                  frame True {
                    w67 = 1 ("Smoothing window")
                    n37 = Get Date/Time In Seconds() -> (seconds since 1Jan1904=w83:timestamp)
                    n38 = To Double Precision Float(number=w83) -> (double precision float=w82:dbl)
                    n39 = call "AppendData.vi"("Smoothing window"=w67, "Current Measurement"=w84) -> ("Data Out"=w70:sgl[][])  [unwired: 4 in]
                    n40 = call "AppendData.vi"("Smoothing window"=w67, "Current Measurement"=w74) -> ("Data Out"=w71:sgl[][])  [unwired: 4 in]
                    n41 = call "AppendData.vi"("Smoothing window"=w67, "Current Measurement"=w75) -> ("Data Out"=w72:sgl[][])  [unwired: 4 in]
                    n42 = call "AppendData1.vi"("Smoothing window"=w67, "Current Measurement"=w82) -> ("Data Out"=w65:dbl[])  [unwired: 4 in]
                    n43 = call "AppendData.vi"("Smoothing window"=w67, "Current Measurement"=w68) -> ("Data Out"=w66:sgl[][])  [unwired: 4 in]
                    n44 = call "MultiRPlot_Select1.vi"("Time"=w65, "FP Plots Select"="FP Plots Select", "Data In"=w70) -> ("Out Array"=→"Front Panel":cluster{"Time":dbl[], "Value":dbl[]}[])  [unwired: 1 in]
                    n45 = call "MultiRPlot_Select1.vi"("Time"=w65, "FP Plots Select"="MG Plots Select", "Data In"=w71) -> ("Out Array"=→"MaxiGauge":cluster{"Time":dbl[], "Value":dbl[]}[])  [unwired: 1 in]
                    n46 = call "MultiRPlot_Select1.vi"("Time"=w65, "FP Plots Select"="PT1 Plots Select", "Data In"=w72) -> ("Out Array"=→"PT1 Status 2":cluster{"Time":dbl[], "Value":dbl[]}[])  [unwired: 1 in]
                    n47 = call "MultiRPlot_Select1.vi"("Time"=w65, "FP Plots Select"="PT2 Plots Select", "Data In"=w66) -> ("Out Array"=→"PT2 Status":cluster{"Time":dbl[], "Value":dbl[]}[])  [unwired: 1 in]
                  }
                }
                n48 = Array To Cluster(array=w36) -> (cluster=w62:T20)
                n49 = call <userlib>:"FP_to_DSC.vi"("FP cluster"=w31) -> ()  [unwired: 10 in, 1 out]
                n50 = property on="P8" class="Ring (strict)"() -> ("Value"=w60:u16)  [unwired: 2 in, 2 out]
                n51 = Unbundle(w62) -> ("FP Data[0]"=→"P1" →"P1":sgl, "FP Data[1]"=→"P2" →"P2":sgl, "FP Data[2]"=→"P3" →"P3":sgl, "FP Data[3]"=→"P4" →"P4":sgl, "FP Data[4]"=→"P5" →"P5":sgl, "FP Data[5]"=→"P6" →"4He":sgl, "FP Data[6]"=→"P7" →"3He":sgl, "FP Data[7]"=→"Flow" →"FLOW":sgl, "FP Data[8]"=→"PC" →"PC":sgl)
                n52 = Index Array(array=w35, index=w60) -> (element=→"Pstill (P8)":dbl)
              }
              frame #1 {
                # "Check if the structure is \nnot empty and only one\nof Scalar or Array controls \nis set"
                # "Set FP control value from external script/program"
                n53 = local read "SetControl"() -> (w125:T7)
                n54 = Unbundle By Name(w125) -> ("Name"=w123:string, "Scalar"=w124:string, "Array"=w115:string[][])
                n55 = call <userlib>:"Empty 2D Array (String)__ogtk.vi"("Array"=w115) -> ("Empty Array?"=w118:bool)  [unwired: 8 in]
                n56 = Empty String/Path?(string/path=w123) -> (empty?=w119:bool)
                n57 = Empty String/Path?(string/path=w124) -> (empty?=w120:bool)
                n58 = Not(x=w119) -> (.not. x?=w121:bool)
                n59 = Not(x=w120) -> (.not. x?=w117:bool)
                n60 = Not(x=w118) -> (.not. x?=w114:bool)
                n61 = Exclusive Or(1:w114, 2:w117) -> (0:w116:bool)
                n62 = And(x=w121, y=w116) -> (x .and. y?=w122:bool)
                n63 = case shown="True" w122 {
                  tunnel: w123 -> [_ w129]
                  tunnel: w124 -> [_ w128]
                  tunnel: w115 -> [_ w127]
                  tunnel: w114 -> [_ w126]
                  frame False {
                  }
                  frame True {
                    n64 = flat-sequence {
                      tunnel: w129 -> [w133]
                      tunnel: w128 -> [w132]
                      tunnel: w127 -> [w130]
                      tunnel: w126 -> [w131]
                      frame #0 {
                        n65 = local read "VIRef"() -> (w134:T1)
                        n66 = case shown="True" w131 {
                          tunnel: w134 -> [w137 w140]
                          tunnel: w133 -> [w136 w139]
                          tunnel: w132 -> [w135 _]
                          tunnel: w130 -> [_ w138]
                          frame False {
                            n67 = call "Push2VI.vi"("New Value"=w135, "element"=w136, "VIRef"=w137) -> ()  [unwired: 8 in, 1 out]
                          }
                          frame True {
                            n68 = call "PushArray2VI.vi"("Str"=w138, "element"=w139, "VIRef"=w140) -> ()  [unwired: 8 in, 1 out]
                          }
                        }
                      }
                      frame #1 {
                        w142 = ""
                        # "Empty the cluster to flag that\nthe command is processed"
                        n69 = Bundle(w142, w142, "Array"=string[][] []) -> (→"SetControl":cluster{string, string, "Array":string[][]})  [unwired: 1 in]
                      }
                    }
                  }
                }
              }
              frame #2 {
                n70 = case shown="True" "EnableAutoCond" {
                  tunnel: w145 -> [w147 w163]
                  tunnel: [w147 w162] -> w144
                  frame False {
                    n71 = call "MGI Milliseconds Since Last Reset.vi"("Reset (F)"=TRUE) -> ()  [unwired: 5 in, 2 out]
                  }
                  frame True {
                    n72 = local read "MG Data"() -> (w170:dbl[])
                    n73 = Index Array(array=w170, index="MG  channel") -> (element=w168:dbl)
                    n74 = Not(x="Cond2") -> (.not. x?=w164:bool)
                    n75 = Less?(x=w168, y="P threshold") -> (x < y?=w166:bool)
                    n76 = Or(x=w166, y=w164) -> (x .or. y?=w150:bool)
                    "SP reached? 3" <- w150
                    n77 = Not(x=w150) -> (.not. x?=w152:bool)
                    n78 = call "MGI Milliseconds Since Last Reset.vi"("Reset (F)"=w152) -> ("ms"=w161:u32)  [unwired: 5 in, 1 out]
                    n79 = Divide(x=w161, y=u32 1000) -> (x/y=w158:dbl)
                    "Delay Timer" <- w158
                    n80 = Multiply(x="Delay Time", y=u32 60) -> (x*y=w154:u32)
                    n81 = Not(x="Cond1") -> (.not. x?=w155:bool)
                    n82 = Greater Or Equal?(x=w158, y=w154) -> (x >= y?=w157:bool)
                    n83 = Or(x=w157, y=w155) -> (x .or. y?=w151:bool)
                    "SP reached? 2" <- w151
                    n84 = And(x=w150, y=w151) -> (x .and. y?=w149:bool)
                    "SP reached?" <- w149
                    n85 = case shown="True" w149 {
                      tunnel: w163 -> [w171 w173]
                      tunnel: [w171 w172] -> w162
                      frame False {
                      }
                      frame True {
                        # "Auto"
                        # "Start"
                        # "Reset"
                        n86 = call "BP togglekey.vi"("keynumber"=u16 10, "FrontPanel port"=w173) -> ("error out"=w185:T19, "FrontPanel port"=w180:refnum<visa-resource-name>)  [unwired: 2 in]
                        n87 = local write "EnableAutoCond"(FALSE ("EnableAutoCond")) -> ()
                        n88 = call "MGI Wait (U32).vi"("ms"=u32 2000, "Error In"=w185) -> ("Error Out"=w184:errorcluster)  [unwired: 5 in]
                        n89 = call "BP togglekey.vi"("error in"=w184, "keynumber"=u16 48, "FrontPanel port"=w180) -> ("error out"=w183:T19, "FrontPanel port"=w182:refnum<visa-resource-name>)  [unwired: 1 in]
                        n90 = call "MGI Wait (U32).vi"("ms"=u32 500, "Error In"=w183) -> ("Error Out"=w181:errorcluster)  [unwired: 5 in]
                        n91 = call "BP togglekey.vi"("error in"=w181, "keynumber"=u16 54, "FrontPanel port"=w182) -> ("FrontPanel port"=w172:refnum<visa-resource-name>)  [unwired: 1 in, 1 out]
                      }
                    }
                  }
                }
              }
            }
          }
          frame True {
            n92 = stacked-sequence {
              frame #0 {
                w191 = T21."Page Disabled & Grayed" ("Page Enabled State")
                w192 = u8 2 ("Disabled")
                w205 = u8 1 ("Disabled")
                w209 = u32 16777062
                w214 = u32 65382
                w213 = u32 0
                w212 = 0.1
                w211 = 2000
                w210 = 0
                n93 = property class="App"() -> ("App.Kind"=w215:T22)  [unwired: 2 in, 2 out]
                n94 = property on="Hide side panel" class="Bool (strict)"("Val(Sgnl)"=FALSE ("Value (Signaling)")) -> ()  [unwired: 2 in, 2 out]
                n95 = property on="S1" class="TabCtl (strict)"("Disabled"=w192) -> ()  [unwired: 2 in, 2 out]
                n96 = property on="S2" class="TabCtl (strict)"("Disabled"=w192) -> ()  [unwired: 2 in, 2 out]
                n97 = property on="Stop" class="Bool (strict)"("Disabled"=w192) -> ()  [unwired: 2 in, 2 out]
                n98 = property on="Error panel" class="TabCtl (strict)"("Disabled"=w192) -> ()  [unwired: 2 in, 2 out]
                n99 = property on="Main Panel" class="TabCtl (strict)"("Disabled"=w192) -> ()  [unwired: 2 in, 2 out]
                n100 = property on="Main Panel" class="TabCtl (strict)"("Disabled"=w192) -> ()  [unwired: 2 in, 2 out]
                n101 = call <userlib>:"Current VIs Reference__ogtk.vi"() -> ("Current VI's reference"=w199:refnum<vi>)  [unwired: 5 in]
                n102 = case shown="\"invalid app kind\", Default" w215 {
                  tunnel: [w217 w226] -> w216
                  frame "invalid app kind", Default {
                    n103 = control-ref of="This VI"() -> (w218:refnum<vi>)
                    n104 = property class="VI"(reference=w218) -> ("Hist.Revision"=w219:u32)  [unwired: 1 in, 2 out]
                    n105 = Divide(x=w219, y=1000.0 ("x")) -> (x/y=w223:dbl)
                    n106 = Number To Fractional String(use system decimal point (T)=FALSE, number=w223, precision (6)=i16 2) -> (F-format string=w224:string)  [unwired: 1 in]
                    n107 = Concatenate Strings("" ("string"), w224) -> (w217:string)
                  }
                  frame "Run Time System" {
                    n108 = Current VI's Path() -> (path=w229:path)
                    n109 = Strip Path(path=w229) -> (stripped path=w230:path)  [unwired: 1 out]
                    n110 = Path To String(path=w230) -> (string=w228:string)
                    n111 = invoke class="FileVersionInfo" method="GetVersionInfo"("fileName"=w228) -> ("GetVersionInfo"=w227:refnum<k24>)  [unwired: 3 in, 3 out]
                    n112 = property class="FileVersionInfo"(reference=w227) -> ("FileVersion"=w226:string)  [unwired: 1 in, 2 out]
                  }
                }
                "V" <- w216
                n113 = local write "Cur Path"(path "") -> ()
                n114 = call "GetFrontPanelControls.vi"("Ref to VI"=w199) -> ("VIRef"=w200:T1)  [unwired: 9 in, 1 out]
                "VIRef" <- w200
                n115 = Unbundle By Name(w200) -> ("Full Name"=→"ControlNames":string[])
                n116 = property on="Side Panel" class="TabCtl (strict)"("Value"=enum32{"Main", "Settings", "Advanced"}."Settings" ("Side Panel")) -> ("Pages"=w188:refnum<vi>[])  [unwired: 2 in, 2 out]
                n117 = Index Array(array=w188) -> (element #1=w189:refnum<vi>, element #3=w190:refnum<vi>)  [unwired: 3 in, 1 out]
                n118 = property class="Page"(reference=w189, "PageEnb"=w191) -> ()  [unwired: 1 in, 2 out]
                n119 = property class="Page"(reference=w190, "PageEnb"=w191) -> ()  [unwired: 1 in, 2 out]
                n120 = property on="3He" class="Slide (strict)"("Scale.Range:Minimum"=w210, "Scale.Range:Maximum"=w211, "Scale.Range:Increment"=w212) -> ()  [unwired: 2 in, 2 out]
                n121 = property on="P1" class="DigNum (strict)"("Numeric Text.Text Colors:Text Color"=w213, "Numeric Text.Text Colors:BG Color"=w209) -> ()  [unwired: 2 in, 2 out]
                n122 = property on="P4" class="DigNum (strict)"("Numeric Text.Text Colors:Text Color"=w213, "Numeric Text.Text Colors:BG Color"=w214) -> ()  [unwired: 2 in, 2 out]
                n123 = Initialize Array(FALSE, 64 ("dimension size")) -> (w193:bool[])
                n124 = property on="Start" class="Bool (strict)"("Visible"=TRUE, "Disabled"=u8 0) -> ()  [unwired: 2 in, 2 out]
                n125 = control-ref of="LEDs"() -> (w196:refnum<vi>)
                n126 = call "FP Set Binking Controls.vi"("Cluster in"=w196, "Array of blinking states"=w193) -> ()  [unwired: 5 in]
                n127 = property on="P2" class="DigNum (strict)"("Numeric Text.Text Colors:Text Color"=w213, "Numeric Text.Text Colors:BG Color"=w209) -> ()  [unwired: 2 in, 2 out]
                n128 = property on="P5" class="DigNum (strict)"("Numeric Text.Text Colors:Text Color"=w213, "Numeric Text.Text Colors:BG Color"=w214) -> ()  [unwired: 2 in, 2 out]
                n129 = property on="4He" class="Slide (strict)"("Scale.Range:Minimum"=w210, "Scale.Range:Maximum"=w211, "Scale.Range:Increment"=w212) -> ()  [unwired: 2 in, 2 out]
                n130 = control-ref of="LEDs 2"() -> (w197:refnum<vi>)
                n131 = property on="Configuration" class="Clust (strict)"("Disabled"=u8 0) -> ()  [unwired: 2 in, 2 out]
                n132 = call "FP Set Binking Controls.vi"("Cluster in"=w197, "Array of blinking states"=w193) -> ()  [unwired: 5 in]
                n133 = local write "EnableAutoCond"(FALSE ("EnableAutoCond")) -> ()
                n134 = property on="P3" class="DigNum (strict)"("Numeric Text.Text Colors:Text Color"=w213, "Numeric Text.Text Colors:BG Color"=w209) -> ()  [unwired: 2 in, 2 out]
                n135 = property on="FLOW" class="DigNum (strict)"("Numeric Text.Text Colors:Text Color"=w213, "Numeric Text.Text Colors:BG Color"=w214) -> ()  [unwired: 2 in, 2 out]
                n136 = property on="Panel ID" class="Str"("Text.Text Colors:Text Color"=u32 13311) -> ()  [unwired: 2 in, 2 out]
                n137 = property on="Buttons" class="Clust"("Disabled"=w205) -> ()  [unwired: 2 in, 2 out]
                n138 = property on="Buttons 2" class="Clust"("Disabled"=w205) -> ()  [unwired: 2 in, 2 out]
              }
              frame #1 {
                (unwired) T23."HKEY_CURRENT_USER" ("root key (HKEY_LOCAL_MACHINE) 2")
                n139 = control-ref of="Configuration"() -> (w234:refnum<vi>)
                n140 = control-ref of="ADC scaling"() -> (w231:refnum<vi>)
                n141 = Build Array(w234, w231) -> (w236:refnum<vi>[])
                n142 = call <userlib>:"Current VIs Parent Directory__ogtk.vi"("Relative path (.)"=path "config.ini") -> ("Parent Directory (+ Relative)"=w232:path)  [unwired: 4 in]
                n143 = call "Save Load Settings to File by Ref with path.vi"("Array of Cluster References"=w236, "subkey"="SOFTWARE\\Leiden Cryogenics\\FP" ("subkey 2"), "Action"=enum8{"Load", "Save"}."Load", "configuration file path"=w232) -> ()  [unwired: 5 in, 1 out]
              }
            }
          }
        }
      }
      event "Start": Value Change {
        n144 = event-data() -> ()  [unwired: 1 in, 6 out]
        n145 = stacked-sequence {
          tunnel: w246 -> [w251 _ _ _ _]
          tunnel: [w250 _ _ _ _] -> w245
          tunnel: w244 -> [_ w306 _ _ _]
          tunnel: [_ w288 _ _ _] -> w243
          tunnel: w242 -> [_ _ _ _ w342]
          tunnel: w241 -> [_ _ w324 _ _]
          tunnel: w240 -> [_ _ w323 _ _]
          tunnel: [_ _ w319 _ _] -> w239
          tunnel: [_ _ w322 _ _] -> w238
          frame #0 {
            w253 = T19 {"error"=FALSE, "code"=0, "source"=""}  # No error
            n146 = property on="MG Enabled?" class="Bool (strict)"() -> ("Value"=w252:bool)  [unwired: 2 in, 2 out]
            n147 = case shown="True" w252 {
              tunnel: [w256 w269] -> w249
              tunnel: [w254 w267] -> w250
              tunnel: w253 -> [w256 w258]
              tunnel: [FALSE TRUE] -> _
              tunnel: w251 -> [w254 w260]
              frame False {
                # "MaxiGauge not connected"
              }
              frame True {
                w265 = TRUE  # query ID
                w264 = FALSE  # reset MG
                n148 = call "VISA Check port.vi"("error in (no error)"=w258, "VISA Resource Name in"=w260) -> ("error out"=w257:errorcluster, "VISA Resource Name out"=w259:refnum<visa-resource-name>)  [unwired: 8 in]
                n149 = call "MG initialize.vi"("error in (no error)"=w257, "MG query errorstatus"=w264, "ID query"=w265, "MaxiGauge port"=w259) -> ("error out"=w270:errorcluster, "program ID"=→"Maxigauge ID":string, "MaxiGauge port"=w268:refnum<visa-resource-name>)  [unwired: 2 in]
                n150 = call "MG Get Channels Labels.vi"("MaxiGauge port"=w268, "error out 2"=w270) -> ("Array"=w263:string[], "MaxiGauge port"=w267:refnum<visa-resource-name>, "error out"=w269:errorcluster)
                n151 = Array To Cluster(array=w263) -> (cluster=→"Cluster":T24)
                n152 = for {
                  tunnel: w263 -> [w273] mode=indexing
                  i -> [w274]
                  n153 = property on="MaxiGauge" class="XYGraph (strict)"("Active Plot"=w274, "Plot.Plot Name"=w273) -> ()  [unwired: 2 in, 2 out]
                }
                n154 = Search 1D Array(1D array=w263, element="STIL") -> (index of element=w261:i32)  [unwired: 1 in]
                n155 = property on="MG  channel P8" class="Ring (strict)"("Val(Sgnl)"=w261) -> ()  [unwired: 2 in, 2 out]
              }
            }
            "MG error" <- w249
          }
          frame #1 {
            n156 = property on="FP baud rate" class="DigNum (strict)"() -> ("Value"=w275:u32)  [unwired: 2 in, 2 out]
            n157 = call "VISA Check port.vi"("error in (no error)"=T19 {"error"=FALSE, "code"=0, "source"=""} ("error in"), "VISA Resource Name in"=w306) -> ("error out"=w303:errorcluster, "VISA Resource Name out"=w305:refnum<visa-resource-name>)  [unwired: 8 in]
            n158 = call "BP Initialize.vi"("FP baud rate"=w275, "error in (no error)"=w303, "FrontPanel port"=w305) -> ("error out"=w317:errorcluster, "FrontPanel port"=w318:refnum<visa-resource-name>)  [unwired: 4 in]
            n159 = call "BP Get ID.vi"("error in (no error)"=w317, "FrontPanel port"=w318) -> ("error out"=w277:errorcluster, "Device ID string"=w283:string, "FrontPanel port"=w316:refnum<visa-resource-name>)  [unwired: 6 in, 1 out]
            "Panel ID" <- w283
            n160 = call "Get GHS version and type.vi"("ID string"=w283, "error in (no error)"=w277) -> ("Panel Version"=w282:bool, "System Type"=w280:bool, "error out"=w276:errorcluster)  [unwired: 4 in]
            n161 = Boolean To (0,1)(Boolean=w282) -> (0, 1=w281:i16)
            n162 = Boolean To (0,1)(Boolean=w280) -> (0, 1=w279:i16)
            n163 = property on="FP Layout" class="TabCtl (strict)"("Value"=w281) -> ()  [unwired: 2 in, 2 out]
            n164 = property on="Type" class="RadioBtnsControl (strict)"("Val(Sgnl)"=w279) -> ()  [unwired: 2 in, 2 out]
            n165 = call "BP query settings.vi"("error in"=w276, "FrontPanel port"=w316) -> ("error out"=w278:T19, "array of 4 x 16 bit unsigned"=w291:u16[], "FrontPanel port"=w292:refnum<visa-resource-name>)  [unwired: 3 in]
            "FP error" <- w278
            n166 = Array To Cluster(array=w291) -> (cluster=w290:T25)
            n167 = call "BP query P5.vi"("error in"=w278, "FrontPanel port"=w292) -> ("error out"=w309:T19, "array of 2 x 16 bit unsigned"=w314:u16[], "FrontPanel port"=w315:refnum<visa-resource-name>)  [unwired: 3 in]
            n168 = property on="P6&7 limits" class="Clust (strict)"("Value"=w290) -> ()  [unwired: 2 in, 2 out]
            n169 = Array To Cluster(array=w314) -> (cluster=w307:T26)
            n170 = call "Disable on error.vi"("error out"=w309) -> ("Numeric"=w310:i16)
            n171 = call "BP query NCP5.vi"("error in"=w278, "FrontPanel port"=w315) -> ("error out"=w312:T19, "array of 3 x 16 bit unsigned"=w313:u16[], "FrontPanel port"=w302:refnum<visa-resource-name>)  [unwired: 3 in]
            n172 = property on="P5 Settings" class="Clust (strict)"("Value"=w307, "Disabled"=w310) -> ()  [unwired: 2 in, 2 out]
            n173 = Array To Cluster(array=w313) -> (cluster=w308:T27)
            n174 = call "Disable on error.vi"("error out"=w312) -> ("Numeric"=w311:i16)
            n175 = call "BP query NCP5B.vi"("error in"=w278, "FrontPanel port"=w302) -> ("error out"=w299:T19, "array of 3 x 16 bit unsigned"=w300:u16[], "FrontPanel port"=w301:refnum<visa-resource-name>)  [unwired: 3 in]
            n176 = property on="P6&7 Settings" class="Clust (strict)"("Value"=w290) -> ()  [unwired: 2 in, 2 out]
            n177 = property on="NCP5 Settings" class="Clust (strict)"("Value"=w308, "Disabled"=w311) -> ()  [unwired: 2 in, 2 out]
            n178 = Array To Cluster(array=w300) -> (cluster=w297:cluster{"array of 3 x 16 bit unsigned[0]":u16})
            n179 = call "Disable on error.vi"("error out"=w299) -> ("Numeric"=w298:i16)
            n180 = call "BP Query REC.vi"("error in"=w278, "FrontPanel port"=w301) -> ("error out"=w295:T19, "array of 3 x 16 bit unsigned"=w296:u16[], "FrontPanel port"=w289:refnum<visa-resource-name>)  [unwired: 3 in]
            n181 = property on="P5 limits" class="Clust (strict)"("Value"=w307) -> ()  [unwired: 2 in, 2 out]
            n182 = property on="NCP5B Settings" class="Clust (strict)"("Value"=w297, "Disabled"=w298) -> ()  [unwired: 2 in, 2 out]
            n183 = Array To Cluster(array=w296) -> (cluster=w293:T27)
            n184 = call "Disable on error.vi"("error out"=w295) -> ("Numeric"=w294:i16)
            n185 = call "BP Query Turbo.vi"("error in"=w278, "FrontPanel port"=w289) -> ("error out"=w286:T19, "array of 3 x 16 bit unsigned"=w285:u16[], "FrontPanel port"=w288:refnum<visa-resource-name>)  [unwired: 3 in]
            n186 = property on="REC Settings" class="Clust (strict)"("Value"=w293, "Disabled"=w294) -> ()  [unwired: 2 in, 2 out]
            n187 = property on="NCP5 limits" class="Clust (strict)"("Value"=w308) -> ()  [unwired: 2 in, 2 out]
            n188 = Array To Cluster(array=w285) -> (cluster=w284:cluster{"array of 3 x 16 bit unsigned[0]":u16})
            n189 = call "Disable on error.vi"("error out"=w286) -> ("Numeric"=w287:i16)
            n190 = property on="S1&2 Settings" class="Clust (strict)"("Value"=w284, "Disabled"=w287) -> ()  [unwired: 2 in, 2 out]
            n191 = property on="NCP5B limits" class="Clust (strict)"("Value"=w297) -> ()  [unwired: 2 in, 2 out]
            n192 = property on="REC limits" class="Clust (strict)"("Value"=w293) -> ()  [unwired: 2 in, 2 out]
            n193 = property on="S1&2 limits" class="Clust (strict)"("Value"=w284) -> ()  [unwired: 2 in, 2 out]
          }
          frame #2 {
            n194 = property on="S2 Enabled?" class="Bool (strict)"() -> ("Value"=w320:bool)  [unwired: 2 in, 2 out]
            n195 = property on="S1 Enabled?" class="Bool (strict)"() -> ("Value"=w321:bool)  [unwired: 2 in, 2 out]
            n196 = case shown="False" w321 {
              tunnel: w324 -> [w328 w330]
              tunnel: [w328 w329] -> w319
              frame False {
              }
              frame True {
                n197 = call "PV Initialize.vi"("VISA session in"=w330) -> ("VISA session out"=w329:refnum<visa-resource-name>)  [unwired: 9 in, 1 out]
              }
            }
            n198 = case shown="False" w320 {
              tunnel: w323 -> [w325 w327]
              tunnel: [w325 w326] -> w322
              frame False {
              }
              frame True {
                n199 = call "PV Initialize.vi"("VISA session in"=w327) -> ("VISA session out"=w326:refnum<visa-resource-name>)  [unwired: 9 in, 1 out]
              }
            }
          }
          frame #3 {
            w335 = T21."Page Enabled" ("Page Enabled State")
            w336 = u8 0 ("Disabled")
            w339 = u8 0 ("Disabled")
            n200 = property on="Configuration" class="Clust (strict)"("Disabled"=u8 2) -> ()  [unwired: 2 in, 2 out]
            n201 = property on="Buttons" class="Clust"("Disabled"=w339) -> ()  [unwired: 2 in, 2 out]
            n202 = property on="Buttons 2" class="Clust"("Disabled"=w339) -> ()  [unwired: 2 in, 2 out]
            n203 = local write "Start"(FALSE ("Start")) -> ()
            n204 = property on="Main Panel" class="TabCtl (strict)"("Disabled"=w336) -> ()  [unwired: 2 in, 2 out]
            n205 = property on="Main Panel" class="TabCtl (strict)"("Disabled"=w336) -> ()  [unwired: 2 in, 2 out]
            n206 = property on="Stop" class="Bool (strict)"("Disabled"=w336) -> ()  [unwired: 2 in, 2 out]
            n207 = property on="Error panel" class="TabCtl (strict)"("Disabled"=w336) -> ()  [unwired: 2 in, 2 out]
            n208 = property on="Side Panel" class="TabCtl (strict)"("Value"=enum32{"Main", "Settings", "Advanced"}."Main" ("Side Panel")) -> ("Pages"=w332:refnum<vi>[])  [unwired: 2 in, 2 out]
            n209 = Index Array(array=w332) -> (element #1=w333:refnum<vi>, element #3=w334:refnum<vi>)  [unwired: 3 in, 1 out]
            n210 = property class="Page"(reference=w333, "PageEnb"=w335) -> ()  [unwired: 1 in, 2 out]
            n211 = property class="Page"(reference=w334, "PageEnb"=w335) -> ()  [unwired: 1 in, 2 out]
          }
          frame #4 {
            n212 = Set Occurrence(w342) -> ()
            n213 = property on="Start" class="Bool (strict)"("Visible"=TRUE, "Disabled"=u8 2) -> ()  [unwired: 2 in, 2 out]
          }
        }
      }
      event "Stop": Value Change {
        w343 = refnum<visa-resource-name> refnum ("PT port")
        w344 = u8 0
        n214 = event-data() -> ()  [unwired: 1 in, 6 out]
        n215 = flat-sequence {
          tunnel: w345 -> [w351]
          tunnel: w349 -> [w354]
          tunnel: w348 -> [w352]
          tunnel: w347 -> [w353]
          tunnel: w346 -> [w355]
          frame #0 {
            n216 = Wait on Occurrence(2:w351) -> ()  [unwired: 2 in, 1 out]
          }
          frame #1 {
            n217 = VISA Close(VISA resource name=w354) -> ()  [unwired: 1 in, 1 out]
            n218 = VISA Close(VISA resource name=w352) -> ()  [unwired: 1 in, 1 out]
            n219 = VISA Close(VISA resource name=w353) -> ()  [unwired: 1 in, 1 out]
            n220 = VISA Close(VISA resource name=w355) -> ()  [unwired: 1 in, 1 out]
          }
          frame #2 {
            (unwired) T23."HKEY_CURRENT_USER" ("root key (HKEY_LOCAL_MACHINE) 2")
            n221 = control-ref of="ADC scaling"() -> (w356:refnum<vi>)
            n222 = control-ref of="Configuration"() -> (w360:refnum<vi>)
            n223 = Build Array(w360, w356) -> (w362:refnum<vi>[])
            n224 = property on="Start" class="Bool (strict)"("Visible"=TRUE) -> ()  [unwired: 2 in, 2 out]
            n225 = call <userlib>:"Current VIs Parent Directory__ogtk.vi"("Relative path (.)"=path "config.ini") -> ("Parent Directory (+ Relative)"=w358:path)  [unwired: 4 in]
            n226 = call "Save Load Settings to File by Ref with path.vi"("Array of Cluster References"=w362, "subkey"="SOFTWARE\\Leiden Cryogenics\\FP" ("subkey 2"), "Action"=enum8{"Load", "Save"}."Save", "configuration file path"=w358) -> ()  [unwired: 5 in, 1 out]
          }
          frame #3 {
            n227 = property on="Stop" class="Bool (strict)"("Value"=FALSE ("stop")) -> ()  [unwired: 2 in, 2 out]
          }
          frame #4 {
            n228 = Stop(stop? (T)=TRUE) -> ()
          }
        }
      }
      event "PT Start": Value Change {
        w374 = u16 54529 items=["Compressor START"=54529, "Compressor STOP"=50584, "Error Code"=26020, "Reset Max/Min"=54235] ("Command")
        n229 = event-data() -> ()  [unwired: 1 in, 6 out]
        n230 = property on="PT1 Address" class="DigNum (strict)"() -> ("Value"=w367:u8)  [unwired: 2 in, 2 out]
        n231 = property on="PT1 Bauds" class="DigNum (strict)"() -> ("Value"=w366:u32)  [unwired: 2 in, 2 out]
        n232 = call "PT Send Command.vi"("Com Port #"=w371, "PT Address"=w367, "PT Bauds"=w366, "Command"=w374) -> ()  [unwired: 1 in, 2 out]
      }
      event "PT Start 2": Value Change {
        w383 = u16 54529 items=["Compressor START"=54529, "Compressor STOP"=50584, "Error Code"=26020, "Reset Max/Min"=54235] ("Command")
        n233 = event-data() -> ()  [unwired: 1 in, 6 out]
        n234 = property on="PT2 Address" class="DigNum (strict)"() -> ("Value"=w376:u8)  [unwired: 2 in, 2 out]
        n235 = property on="PT2 Bauds" class="DigNum (strict)"() -> ("Value"=w375:u32)  [unwired: 2 in, 2 out]
        n236 = call "PT Send Command.vi"("Com Port #"=w377, "PT Address"=w376, "PT Bauds"=w375, "Command"=w383) -> ()  [unwired: 1 in, 2 out]
      }
      event "PT_stop": Value Change {
        w392 = u16 50584 items=["Compressor START"=54529, "Compressor STOP"=50584, "Error Code"=26020, "Reset Max/Min"=54235] ("Command")
        n237 = event-data() -> ()  [unwired: 1 in, 1 out]
        n238 = property on="PT1 Address" class="DigNum (strict)"() -> ("Value"=w385:u8)  [unwired: 2 in, 2 out]
        n239 = property on="PT1 Bauds" class="DigNum (strict)"() -> ("Value"=w384:u32)  [unwired: 2 in, 2 out]
        n240 = call "PT Send Command.vi"("Com Port #"=w389, "PT Address"=w385, "PT Bauds"=w384, "Command"=w392) -> ()  [unwired: 1 in, 2 out]
      }
      event "PT_stop 2": Value Change {
        w401 = u16 50584 items=["Compressor START"=54529, "Compressor STOP"=50584, "Error Code"=26020, "Reset Max/Min"=54235] ("Command")
        n241 = event-data() -> ()  [unwired: 1 in, 1 out]
        n242 = property on="PT2 Address" class="DigNum (strict)"() -> ("Value"=w394:u8)  [unwired: 2 in, 2 out]
        n243 = property on="PT2 Bauds" class="DigNum (strict)"() -> ("Value"=w393:u32)  [unwired: 2 in, 2 out]
        n244 = call "PT Send Command.vi"("Com Port #"=w395, "PT Address"=w394, "PT Bauds"=w393, "Command"=w401) -> ()  [unwired: 1 in, 2 out]
      }
      event "PT Error Code": Value Change {
        n245 = event-data() -> ("OldVal"=w410:i32, "NewVal"=w406:i32)  [unwired: 1 in]
        n246 = Not Equal?(x=w410, y=w406) -> (x != y?=w409:bool)
        n247 = global read "ErrCodeStatusLkup.vi" "Error code/name/description Firmware V1.5"() -> (w407:string)
        n248 = case shown="Default" w406 {
          tunnel: w408 -> [_ w421]
          frame 0, 14..23 {
            # "No Error or Warning"
            "Attempts Counter" <- u16 0 ("Attempts Counter")
          }
          frame Default {
            # "Error"
            n249 = local read "Attempts Counter"() -> (w427:u16)
            n250 = Less?(x=w427, y="Attempts") -> (x < y?=w424:bool)
            n251 = And(x=w424, y="Restart PT on Error?") -> (x .and. y?=w423:bool)
            n252 = case shown="True" w423 {
              tunnel: "Time delay" -> [_ w429]
              tunnel: w421 -> [_ w428]
              frame False {
              }
              frame True {
                n253 = flat-sequence {
                  tunnel: w428 -> [w430]
                  tunnel: w429 -> [w434]
                  frame #0 {
                    n254 = call "PT start.vi"("Com Port #"=w430) -> ()  [unwired: 1 in, 2 out]
                  }
                  frame #1 {
                    n255 = local read "Attempts Counter"() -> (w432:u16)
                    n256 = Increment(x=w432) -> (x+1=w431:u16)
                    n257 = local write "Attempts Counter"(w431) -> ()
                  }
                  frame #2 {
                    n258 = Multiply(x=w434, y=u16 1000) -> (x*y=w435:u16)
                    n259 = Wait (ms)(milliseconds to wait=w435) -> ()  [unwired: 1 out]
                  }
                }
              }
            }
          }
        }
        n260 = Pick Line(multi-line string=w407, line index=w406) -> (output string=w405:string)  [unwired: 1 in]
        "PT Error" <- w405
        n261 = case shown="True" w409 {
          tunnel: w406 -> [_ w416]
          tunnel: w405 -> [_ w413]
          frame False {
          }
          frame True {
            n262 = Format Date/Time String() -> (date/time string=w414:string)  [unwired: 3 in]
            n263 = Number To Decimal String(number=w416) -> (decimal integer string=w415:string)  [unwired: 1 in]
            n264 = Build Array(w414, w415, w413) -> (w417:string[])
            n265 = feedback #1() -> (w418:string[][])  [unwired: 1 in]
            "Error Log" <- w418
            n266 = Build Array (concatenate)(w418, w417) -> (w419:string[][])
            n267 = feedback-in #1(w419) -> ()
          }
        }
      }
      event "PT_ResetValues": Value Change {
        w444 = u16 54235 items=["Compressor START"=54529, "Compressor STOP"=50584, "Error Code"=26020, "Reset Max/Min"=54235] ("Command")
        n268 = event-data() -> ()  [unwired: 1 in, 1 out]
        n269 = property on="PT1 Address" class="DigNum (strict)"() -> ("Value"=w437:u8)  [unwired: 2 in, 2 out]
        n270 = property on="PT1 Bauds" class="DigNum (strict)"() -> ("Value"=w436:u32)  [unwired: 2 in, 2 out]
        n271 = call "PT Send Command.vi"("Com Port #"=w441, "PT Address"=w437, "PT Bauds"=w436, "Command"=w444) -> ()  [unwired: 1 in, 2 out]
      }
      event "PT_ResetValues 2": Value Change {
        w453 = u16 54235 items=["Compressor START"=54529, "Compressor STOP"=50584, "Error Code"=26020, "Reset Max/Min"=54235] ("Command")
        n272 = event-data() -> ()  [unwired: 1 in, 1 out]
        n273 = property on="PT2 Address" class="DigNum (strict)"() -> ("Value"=w446:u8)  [unwired: 2 in, 2 out]
        n274 = property on="PT2 Bauds" class="DigNum (strict)"() -> ("Value"=w445:u32)  [unwired: 2 in, 2 out]
        n275 = call "PT Send Command.vi"("Com Port #"=w447, "PT Address"=w446, "PT Bauds"=w445, "Command"=w453) -> ()  [unwired: 1 in, 2 out]
      }
      event "Buttons": Value Change {
        n276 = event-data() -> ("NewVal"=w462:T3)  [unwired: 1 in, 5 out]
        n277 = Cluster To Array(cluster=w462) -> (array=w461:bool[])
        n278 = while {
          tunnel: w461 -> [w466] mode=indexing
          tunnel: [w465] -> w460
          i -> [w465]
          stop <- w466 stop-if-true
        }
        n279 = Increment(x=w460) -> (x+1=w459:i32)
        n280 = call "BP togglekey.vi"("keynumber"=w459, "FrontPanel port"=w458) -> ("FrontPanel port"=w457:refnum<visa-resource-name>)  [unwired: 2 in, 1 out]
      }
      event "Buttons 2": Value Change {
        n281 = event-data() -> ("NewVal"=w475:T3)  [unwired: 1 in, 5 out]
        n282 = Cluster To Array(cluster=w475) -> (array=w474:bool[])
        n283 = while {
          tunnel: w474 -> [w479] mode=indexing
          tunnel: [w478] -> w473
          i -> [w478]
          stop <- w479 stop-if-true
        }
        n284 = Increment(x=w473) -> (x+1=w472:i32)
        n285 = call "BP togglekey.vi"("keynumber"=w472, "FrontPanel port"=w471) -> ("FrontPanel port"=w470:refnum<visa-resource-name>)  [unwired: 2 in, 1 out]
      }
      event "Button": Value Change {
        n286 = event-data() -> ()  [unwired: 1 in, 6 out]
        n287 = call "BP togglekey.vi"("keynumber"="Button", "FrontPanel port"=w485) -> ("FrontPanel port"=w484:refnum<visa-resource-name>)  [unwired: 2 in, 1 out]
      }
      event "SET VALUES": Value Change {
        n288 = event-data() -> ("OldVal"=w494:bool)  [unwired: 1 in, 5 out]
        n289 = property on="SET VALUES" class="Bool (strict)"("Value"=w494) -> ()  [unwired: 2 in, 2 out]
        n290 = stacked-sequence {
          tunnel: w489 -> [w500 w512 w525 w541 w554 w567]
          tunnel: [w496 _ _ _ _ _] -> w488
          frame #0 {
            n291 = local read "P6&7 Settings"() -> (w499:T13)
            n292 = local read "P6&7 limits"() -> (w498:T13)
            n293 = Not Equal?(x=w499, y=w498) -> (x != y?=w497:bool)
            n294 = case shown="True" w497 {
              tunnel: w500 -> [w502 w507]
              tunnel: [w502 w506] -> w496
              frame False {
                n295 = control-ref of="P6&7 Settings"() -> (w501:refnum<vi>)
                n296 = call "FP check parameters error.vi"("Clust Refnum"=w501) -> ()  [unwired: 6 in, 1 out]
              }
              frame True {
                n297 = control-ref of="P6&7 Settings"() -> (w503:refnum<vi>)
                n298 = call "BP Set Config.vi"("GHS Settings"="P6&7 Settings", "FrontPanel port"=w507) -> ("error out"=w505:T19, "FrontPanel port"=w511:refnum<visa-resource-name>)  [unwired: 2 in]
                n299 = call "FP check parameters error.vi"("error in"=w505, "Clust Refnum"=w503) -> ("error out"=w504:errorcluster)  [unwired: 5 in]
                n300 = call "BP query settings.vi"("error in"=w504, "FrontPanel port"=w511) -> ("array of 4 x 16 bit unsigned"=w509:u16[], "FrontPanel port"=w506:refnum<visa-resource-name>)  [unwired: 3 in, 1 out]
                n301 = Array To Cluster(array=w509) -> (cluster=→"P6&7 limits":T25)
              }
            }
          }
          frame #1 {
            n302 = local read "P5 Settings"() -> (w514:cluster{"P6 low":u16, "P6 high":u16})
            n303 = local read "P5 limits"() -> (w515:cluster{"P5 C1":u16, "P5 C2":u16})
            n304 = Not Equal?(x=w514, y=w515) -> (x != y?=w513:bool)
            n305 = case shown="True" w513 {
              tunnel: w512 -> [_ w520]
              frame False {
                n306 = control-ref of="P5 Settings"() -> (w516:refnum<vi>)
                n307 = call "FP check parameters error.vi"("Clust Refnum"=w516) -> ()  [unwired: 6 in, 1 out]
              }
              frame True {
                n308 = control-ref of="P5 Settings"() -> (w517:refnum<vi>)
                n309 = call "BP Set P5.vi"("P5 Settings"="P5 Settings", "FrontPanel port in"=w520) -> ("error out"=w524:errorcluster, "FrontPanel port out"=w523:refnum<visa-resource-name>)  [unwired: 2 in]
                n310 = call "FP check parameters error.vi"("error in"=w524, "Clust Refnum"=w517) -> ("error out"=w518:errorcluster)  [unwired: 5 in]
                n311 = call "BP query P5.vi"("error in"=w518, "FrontPanel port"=w523) -> ("array of 2 x 16 bit unsigned"=w522:u16[])  [unwired: 3 in, 2 out]
                n312 = Array To Cluster(array=w522) -> (cluster=→"P5 limits":T26)
              }
            }
          }
          frame #2 {
            n313 = local read "NCP5 Settings"() -> (w527:T10)
            n314 = local read "NCP5 limits"() -> (w528:T12)
            n315 = Not Equal?(x=w527, y=w528) -> (x != y?=w526:bool)
            n316 = case shown="True" w526 {
              tunnel: w525 -> [_ w533]
              frame False {
                n317 = control-ref of="NCP5 Settings"() -> (w529:refnum<vi>)
                n318 = call "FP check parameters error.vi"("Clust Refnum"=w529) -> ()  [unwired: 6 in, 1 out]
              }
              frame True {
                n319 = control-ref of="NCP5 Settings"() -> (w530:refnum<vi>)
                n320 = call "BP Set NCP5.vi"("NCP5 Settings"="NCP5 Settings", "FrontPanel port in"=w533) -> ("error out"=w532:errorcluster, "FrontPanel port out"=w537:refnum<visa-resource-name>)  [unwired: 2 in]
                n321 = call "FP check parameters error.vi"("error in"=w532, "Clust Refnum"=w530) -> ("error out"=w531:errorcluster)  [unwired: 5 in]
                n322 = call "BP query NCP5.vi"("error in"=w531, "FrontPanel port"=w537) -> ("array of 3 x 16 bit unsigned"=w535:u16[])  [unwired: 3 in, 2 out]
                n323 = Array To Cluster(array=w535) -> (cluster=→"NCP5 limits":T27)
              }
            }
          }
          frame #3 {
            n324 = local read "NCP5B Settings"() -> (w538:cluster{"P6 low":u16})
            n325 = local read "NCP5B limits"() -> (w539:cluster{"P5 NC4":u16})
            n326 = Not Equal?(x=w538, y=w539) -> (x != y?=w540:bool)
            n327 = case shown="True" w540 {
              tunnel: w541 -> [_ w546]
              frame False {
                n328 = control-ref of="NCP5B Settings"() -> (w542:refnum<vi>)
                n329 = call "FP check parameters error.vi"("Clust Refnum"=w542) -> ()  [unwired: 6 in, 1 out]
              }
              frame True {
                n330 = control-ref of="NCP5B Settings"() -> (w543:refnum<vi>)
                n331 = call "BP Set NCP5B.vi"("NCP5B"="NCP5B Settings", "FrontPanel port in"=w546) -> ("error out"=w545:errorcluster, "FrontPanel port out"=w547:refnum<visa-resource-name>)  [unwired: 2 in]
                n332 = call "FP check parameters error.vi"("error in"=w545, "Clust Refnum"=w543) -> ("error out"=w544:errorcluster)  [unwired: 5 in]
                n333 = call "BP query NCP5B.vi"("error in"=w544, "FrontPanel port"=w547) -> ("array of 3 x 16 bit unsigned"=w548:u16[])  [unwired: 3 in, 2 out]
                n334 = Array To Cluster(array=w548) -> (cluster=→"NCP5B limits":cluster{"array of 3 x 16 bit unsigned[0]":u16})
              }
            }
          }
          frame #4 {
            n335 = local read "REC Settings"() -> (w552:T10)
            n336 = local read "REC limits"() -> (w553:T11)
            n337 = Not Equal?(x=w552, y=w553) -> (x != y?=w551:bool)
            n338 = case shown="True" w551 {
              tunnel: w554 -> [_ w559]
              frame False {
                n339 = control-ref of="REC Settings"() -> (w555:refnum<vi>)
                n340 = call "FP check parameters error.vi"("Clust Refnum"=w555) -> ()  [unwired: 6 in, 1 out]
              }
              frame True {
                n341 = control-ref of="REC Settings"() -> (w556:refnum<vi>)
                n342 = call "BP Set REC.vi"("NCP5 Settings"="REC Settings", "FrontPanel port in"=w559) -> ("error out"=w558:errorcluster, "FrontPanel port out"=w560:refnum<visa-resource-name>)  [unwired: 2 in]
                n343 = call "FP check parameters error.vi"("error in"=w558, "Clust Refnum"=w556) -> ("error out"=w557:errorcluster)  [unwired: 5 in]
                n344 = call "BP Query REC.vi"("error in"=w557, "FrontPanel port"=w560) -> ("array of 3 x 16 bit unsigned"=w562:u16[])  [unwired: 3 in, 2 out]
                n345 = Array To Cluster(array=w562) -> (cluster=→"REC limits":T27)
              }
            }
          }
          frame #5 {
            n346 = local read "S1&2 Settings"() -> (w564:cluster{"Enum":enum16{"OFF", "ON"}})
            n347 = local read "S1&2 limits"() -> (w565:cluster{"S1&S2":enum16{"OFF", "ON"}})
            n348 = Not Equal?(x=w564, y=w565) -> (x != y?=w566:bool)
            n349 = case shown="True" w566 {
              tunnel: w567 -> [_ w574]
              frame False {
                n350 = control-ref of="S1&2 Settings"() -> (w568:refnum<vi>)
                n351 = call "FP check parameters error.vi"("Clust Refnum"=w568) -> ()  [unwired: 6 in, 1 out]
              }
              frame True {
                n352 = control-ref of="S1&2 Settings"() -> (w569:refnum<vi>)
                n353 = call "BP Set Turbo.vi"("S1&2 Settings"="S1&2 Settings", "FrontPanel port in"=w574) -> ("error out"=w571:errorcluster, "FrontPanel port out"=w575:refnum<visa-resource-name>)  [unwired: 2 in]
                n354 = call "FP check parameters error.vi"("error in"=w571, "Clust Refnum"=w569) -> ("error out"=w570:errorcluster)  [unwired: 5 in]
                n355 = call "BP Query Turbo.vi"("error in"=w570, "FrontPanel port"=w575) -> ("array of 3 x 16 bit unsigned"=w576:u16[])  [unwired: 3 in, 2 out]
                n356 = Array To Cluster(array=w576) -> (cluster=→"S1&2 limits":cluster{"array of 3 x 16 bit unsigned[0]":u16})
              }
            }
          }
        }
      }
      event "Log Options.Plot data": Value Change {
        n357 = event-data() -> ("NewVal"=w583:bool)  [unwired: 1 in, 5 out]
        n358 = property on="Main Panel" class="TabCtl (strict)"() -> ("Pages"=w586:refnum<vi>[])  [unwired: 2 in, 2 out]
        n359 = Index Array(array=w586, index=2) -> (element=w584:refnum<vi>)
        n360 = property class="Page"(reference=w584, "PageVis"=w583) -> ()  [unwired: 1 in, 2 out]
      }
      event "Autoconf": Value Change {
        n361 = event-data() -> ()  [unwired: 1 in, 6 out]
      }
      event "Configuration": Value Change {
        n362 = event-data() -> ()  [unwired: 1 in, 6 out]
        n363 = VISA Close(VISA resource name=w601) -> ()  [unwired: 1 in, 1 out]
        n364 = VISA Close(VISA resource name=w602) -> ()  [unwired: 1 in, 1 out]
        n365 = VISA Close(VISA resource name=w599) -> ()  [unwired: 1 in, 1 out]
        n366 = VISA Close(VISA resource name=w597) -> ()  [unwired: 1 in, 1 out]
        n367 = Unbundle By Name("Configuration") -> ("PT1 port"=w605:refnum<visa-resource-name>, "PT2 port"=w595:refnum<visa-resource-name>, "FP port"=w606:refnum<visa-resource-name>, "MG port"=w600:refnum<visa-resource-name>, "S1 port"=w598:refnum<visa-resource-name>, "S2 port"=w596:refnum<visa-resource-name>)
        n368 = call "VISA to RS232 Port Nr.vi"("VISA Resource Name"=w605) -> ("Port Number"=w604:u8)  [unwired: 1 in]
        n369 = call "VISA to RS232 Port Nr.vi"("VISA Resource Name"=w595) -> ("Port Number"=w593:u8)  [unwired: 1 in]
        n370 = Increment(x=w604) -> (x+1=w603:u8)
        n371 = Increment(x=w593) -> (x+1=w594:u8)
      }
      event "Type": Value Change {
        n372 = event-data() -> ("NewVal"=w611:enum32{"Wet", "CF"})  [unwired: 1 in, 5 out]
        n373 = case shown="\"CF\", Default" w611 {
          tunnel: ["COMPRESSOR" ("Label.Text") "AUX 2" ("Label.Text")] -> w616
          tunnel: [TRUE ("Visible") FALSE ("Visible")] -> w612
          tunnel: ["From\nProbe" ("Text.Text") "From\nDewar" ("Text.Text")] -> w610
          tunnel: ["From\nOVC" ("Text.Text") "From\n1K pot" ("Text.Text")] -> w609
          frame "CF", Default {
          }
          frame "Wet" {
          }
        }
        n374 = property on="Main Panel" class="TabCtl (strict)"() -> ("Pages"=w615:refnum<vi>[])  [unwired: 2 in, 2 out]
        n375 = Index Array(array=w615, index=1) -> (element=w613:refnum<vi>)
        n376 = property on="COMPR/AUX 2" class="Bool (strict)"("Caption.Text"=w616) -> ()  [unwired: 2 in, 2 out]
        n377 = property on="String 3" class="Str"("Text.Text"=w610) -> ()  [unwired: 2 in, 2 out]
        n378 = property on="String" class="Str"("Text.Text"=w609) -> ()  [unwired: 2 in, 2 out]
        n379 = property on="BYPASS" class="Bool (strict)"("Visible"=w612) -> ()  [unwired: 2 in, 2 out]
        n380 = property on="PT STATUS" class="Bool (strict)"("Visible"=w612) -> ()  [unwired: 2 in, 2 out]
        n381 = property class="Page"(reference=w613, "PageVis"=w612) -> ()  [unwired: 1 in, 2 out]
        n382 = property on="String 4" class="Str"("Text.Text"=w610) -> ()  [unwired: 2 in, 2 out]
        n383 = property on="String 2" class="Str"("Text.Text"=w609) -> ()  [unwired: 2 in, 2 out]
      }
      event "FP Status bits": Value Change {
        n384 = event-data() -> ("OldVal"=w638:u32[], "NewVal"=w637:u32[])  [unwired: 1 in, 4 out]
        n385 = Not Equal?(x=w638, y=w637) -> (x != y?=w636:bool)
        n386 = case shown="True" w636 {
          frame False {
          }
          frame True {
            "ForceSave" <- TRUE ("ForceSave")
          }
        }
      }
      event "Front Panel", "MaxiGauge": Shortcut Menu Activation? {
        w644 = string[] ["Log Y"] ("item names")
        w656 = string[] ["Autoscale XY"] ("item names")
        n387 = event-data() -> ("MenuRef"=w642:refnum<k9>, "CtlRef"=w641:refnum<vi>)  [unwired: 1 in]
        n388 = Insert Menu Items(4:10, 7:w656, 8:w656, 9:w642) -> (3:w643:refnum<k9>)  [unwired: 2 in, 2 out]
        n389 = property class="XYGraph (strict)"(reference=w641) -> ("YScale.Mapping Mode"=w647:u8)  [unwired: 1 in, 2 out]
        n390 = Insert Menu Items(4:13, 7:w644, 8:w644, 9:w643) -> (3:w646:refnum<k9>)  [unwired: 2 in, 2 out]
        n391 = Not Equal To 0?(x=w647) -> (x != 0?=w648:bool)
        n392 = Set Menu Item Info(6:w648, 7:"Log Y", 11:w646) -> ()  [unwired: 4 in, 2 out]
        n393 = event-data() -> ()  [unwired: 2 in, 1 out]
      }
      event "Front Panel", "MaxiGauge": Shortcut Menu Selection (User) {
        n394 = event-data() -> ("CtlRef"=w660:refnum<vi>, "ItemTag"=w666:string)  [unwired: 1 in]
        n395 = Type Cast(type=refnum<vi> refnum ("R-Plot 0"), x=w660) -> (*(type *) &x=w659:refnum<vi>)
        n396 = case shown="\"Log Y\"" w666 {
          tunnel: w659 -> [_ w667 w669]
          frame Default {
          }
          frame "Autoscale XY" {
            w668 = u8 2 ("X Scale.Scale Fit")
            n397 = property class="XYGraph (strict)"(reference=w667, "XScale.ScaleFit"=w668, "YScale.ScaleFit"=w668) -> ()  [unwired: 1 in, 2 out]
          }
          frame "Log Y" {
            n398 = property class="XYGraph (strict)"(reference=w669) -> (reference out=w670:refnum<vi>, "YScale.Mapping Mode"=w671:u8)  [unwired: 1 in, 1 out]
            n399 = Equal To 0?(x=w671) -> (x = 0?=w672:bool)
            n400 = Boolean To (0,1)(Boolean=w672) -> (0, 1=w673:i16)
            n401 = property class="XYGraph (strict)"(reference=w670, "YScale.Mapping Mode"=w673) -> ()  [unwired: 1 in, 2 out]
          }
        }
      }
      event "Front Panel", "MaxiGauge": Scale Range Change {
        w681 = u8 0 ("X Scale.Scale Fit")
        n402 = event-data() -> ("CtlRef"=w680:refnum<vi>)  [unwired: 1 in, 7 out]
        n403 = property class="XYGraph (strict)"(reference=w680, "XScale.ScaleFit"=w681, "YScale.ScaleFit"=w681) -> ()  [unwired: 1 in, 2 out]
      }
      event "Reset Error": Value Change {
        n404 = event-data() -> ()  [unwired: 1 in, 6 out]
        n405 = property on="Device address S1" class="DigNum (strict)"() -> ("Value"=w684:u8)  [unwired: 2 in, 2 out]
        n406 = call "PV Error Reset.vi"("Adress of unit"=w684, "VISA session"=w689) -> ("VISA resource out"=w683:refnum<visa-resource-name>)  [unwired: 8 in, 1 out]
      }
      event "Reset Error 2": Value Change {
        n407 = event-data() -> ()  [unwired: 1 in, 6 out]
        n408 = property on="Device address S2" class="DigNum (strict)"() -> ("Value"=w692:u8)  [unwired: 2 in, 2 out]
        n409 = call "PV Error Reset.vi"("Adress of unit"=w692, "VISA session"=w697) -> ("VISA resource out"=w691:refnum<visa-resource-name>)  [unwired: 8 in, 1 out]
      }
      event "Configuration.S1 Enabled?": Value Change {
        n410 = event-data() -> ("NewVal"=w708:bool)  [unwired: 1 in, 5 out]
        n411 = Not(x=w708) -> (.not. x?=w707:bool)
        n412 = Boolean To (0,1)(Boolean=w707) -> (0, 1=w706:i16)
        n413 = Multiply(x=i16 2, y=w706) -> (x*y=w704:i16)
        n414 = property on="S1" class="TabCtl (strict)"("Disabled"=w704) -> ()  [unwired: 2 in, 2 out]
      }
      event "Configuration.S2 Enabled?": Value Change {
        n415 = event-data() -> ("NewVal"=w716:bool)  [unwired: 1 in, 5 out]
        n416 = Not(x=w716) -> (.not. x?=w719:bool)
        n417 = Boolean To (0,1)(Boolean=w719) -> (0, 1=w718:i16)
        n418 = Multiply(x=i16 2, y=w718) -> (x*y=w715:i16)
        n419 = property on="S2" class="TabCtl (strict)"("Disabled"=w715) -> ()  [unwired: 2 in, 2 out]
      }
      event "Boolean 2": Value Change {
        n420 = event-data() -> ("NewVal"=w726:bool)  [unwired: 1 in, 5 out]
        n421 = case shown="False" w726 {
          frame True {
            n422 = property class="VI"() -> ("Front Panel.PanelBounds"=w727:T28)  [unwired: 2 in, 2 out]
            n423 = Unbundle By Name(w727) -> ("Left"=w733:i16, "Top"=w730:i16)
            n424 = Add(x=i16 955 ("right"), y=w733) -> (x+y=w732:i16)
            n425 = Add(x=w730, y=i16 730) -> (x+y=w728:i16)
            n426 = Bundle By Name(cluster=w727, "Right"=w732, "Bottom"=w728) -> (w734:T28)
            n427 = property class="VI"("Front Panel.PanelBounds"=w734) -> ()  [unwired: 2 in, 2 out]
          }
          frame False {
            n428 = property class="VI"() -> ("Front Panel.PanelBounds"=w735:T28)  [unwired: 2 in, 2 out]
            n429 = Unbundle By Name(w735) -> ("Left"=w741:i16, "Top"=w738:i16)
            n430 = Add(x=i16 1259 ("right"), y=w741) -> (x+y=w740:i16)
            n431 = Add(x=w738, y=i16 730) -> (x+y=w736:i16)
            n432 = Bundle By Name(cluster=w735, "Right"=w740, "Bottom"=w736) -> (w742:T28)
            n433 = property class="VI"("Front Panel.PanelBounds"=w742) -> ()  [unwired: 2 in, 2 out]
          }
        }
      }
      event "SendCMD": Value Change {
        n434 = event-data() -> ()  [unwired: 1 in, 6 out]
        n435 = call "BP Send Command.vi"("String"="Command", "FrontPanel port in"=w746) -> ("string after ack"=→"Response":string, "FrontPanel port out"=w745:refnum<visa-resource-name>)  [unwired: 1 in, 1 out]
      }
    }
  }
  n436 = flat-sequence {
    tunnel: w4 -> [w752]
    tunnel: w2 -> [w952]
    frame #0 {
      n437 = Wait on Occurrence(2:w752) -> ()  [unwired: 2 in, 1 out]
    }
    frame #1 {
      n438 = local read "FP error"() -> (w761:errorcluster)
      n439 = property on="PT1 Enabled?" class="Bool (strict)"() -> ("Value"=w767:bool)  [unwired: 2 in, 2 out]
      n440 = property on="FP port" class="VISAName"() -> ("Value"=w763:refnum<visa-resource-name>)  [unwired: 2 in, 2 out]
      n441 = property on="PT1 Bauds" class="DigNum (strict)"() -> ("Value"=w765:u32)  [unwired: 2 in, 2 out]
      n442 = property on="PT1 \nAddress" class="DigNum (strict)"() -> ("Value"=w768:u8)  [unwired: 2 in, 2 out]
      n443 = property on="PT1 port" class="VISAName"() -> ("Value"=w771:refnum<visa-resource-name>)  [unwired: 2 in, 2 out]
      n444 = call "VISA to RS232 Port Nr.vi"("VISA Resource Name"=w771) -> ("Port Number"=w770:u8)  [unwired: 1 in]
      n445 = Increment(x=w770) -> (x+1=w769:u8)
      n446 = while {
        shift-right: [w816] -> _
        shift-left: w761 -> [w817]
        shift-right: [w814] -> _
        shift-left: w763 -> [w815]
        stop <- "Stop" stop-if-true
        # "Front Panel"
        n447 = case shown="No Error" w817 {
          selector: w817 -> [w850 _]
          tunnel: [w825 w859] -> w814
          tunnel: [w823 w857] -> w816
          tunnel: w815 -> [w851 w860]
          frame No Error {
            n448 = call "BP Query KeyStatus.vi"("error in"=w850, "FrontPanel port"=w851) -> ("error out"=w835:T19, "Button states"=w849:bool[], "Blinking States"=w821:bool[], "FrontPanel port"=w836:refnum<visa-resource-name>)  [unwired: 2 in]
            n449 = property on="Pstill (P8)" class="DigNum (strict)"() -> ("Value"=w837:dbl)  [unwired: 2 in, 2 out]
            n450 = property on="AutoStop" class="Bool (strict)"() -> ("Value"=w838:bool)  [unwired: 2 in, 2 out]
            n451 = call "BP Query Status.vi"("error in"=w835, "FrontPanel port"=w836) -> ("error out"=w840:T19, "status word (32 bit unsigned)"=w843:u32, "FrontPanel port"=w841:refnum<visa-resource-name>)  [unwired: 3 in]
            n452 = Build Array (concatenate)(w849, FALSE) -> (w847:bool[])
            n453 = call "FP encode still pressure.vi"("Value 2"=w838, "Value"=w837) -> ("Numeric"=w842:u16)  [unwired: 4 in]
            n454 = Array To Cluster(array=w847) -> (cluster=→"LEDs" →"LEDs 2":T29)
            n455 = call "FP decode mode & alarm.vi"("status word (32 bit unsigned)"=w843) -> ("Boolean"=w839:bool, "Numeric"=→"Mode":u32)  [unwired: 4 in]
            n456 = call "FP status from bits to numeric.vi"("FP Status bits"=w847) -> ("FP status number"=w846:u32[])  [unwired: 4 in]
            n457 = call "BP Send Values.vi"("error in"=w840, "value to send"=w842, "FrontPanel port"=w841) -> ("error out"=w828:T19, "FrontPanel port"=w829:refnum<visa-resource-name>)  [unwired: 3 in]
            n458 = property on="FP Status bits" class="Arr (strict)"("Val(Sgnl)"=w846) -> ()  [unwired: 2 in, 2 out]
            n459 = property on="P5 alarm" class="Bool (strict)"("Blinking"=w839, "Value"=w839) -> ()  [unwired: 2 in, 2 out]
            n460 = call "BP Query Adc.vi"("error in"=w828, "FrontPanel port"=w829) -> ("error out"=w824:T19, "array of 8(9) x 16 bit unsigned"=w827:i32[], "FrontPanel port"=w825:refnum<visa-resource-name>)  [unwired: 3 in]
            n461 = Cluster To Array(cluster="ADC scaling") -> (array=w826:dbl[])
            n462 = call "BP Scale Adc-NEW PANEL.vi"("input array scaling factors,8(9) x 16 bit uint"=w826, "input array 8(9) x 16bit uint"=w827) -> ("output array 8(9) x single prec. incl flow"=w834:sgl[])  [unwired: 4 in, 1 out]
            n463 = property on="Averages" class="DigNum (strict)"() -> ("Value"=w833:i32)  [unwired: 2 in, 2 out]
            n464 = control-ref of="LEDs"() -> (w820:refnum<vi>)
            n465 = call "FP Set Binking Controls.vi"("Cluster in"=w820, "Array of blinking states"=w821) -> ()  [unwired: 5 in]
            n466 = call "Running average.vi"("Window Size"=w833, "New values"=w834, "Filter Zeroes? (T)"=FALSE) -> ("Filterred"=→"FP Data":dbl[])  [unwired: 1 in]
            n467 = control-ref of="LEDs 2"() -> (w819:refnum<vi>)
            n468 = call "FP Set Binking Controls.vi"("Cluster in"=w819, "Array of blinking states"=w821) -> ()  [unwired: 5 in]
            n469 = call <userlib>:"Wait (ms)__ogtk.vi"("error in (no error)"=w824, "milliseconds to wait"=u32 250) -> ("error out"=w823:errorcluster)  [unwired: 8 in, 1 out]
          }
          frame Error {
            n470 = property on="FP baud rate" class="DigNum (strict)"() -> ("Value"=w852:u32)  [unwired: 2 in, 2 out]
            n471 = VISA Close(VISA resource name=w860) -> (error out=w869:errorcluster)  [unwired: 1 in]
            n472 = call "VISA Check port.vi"("error in (no error)"=w869, "VISA Resource Name in"=w860) -> ("error out"=w868:errorcluster, "VISA Resource Name out"=w867:refnum<visa-resource-name>)  [unwired: 8 in]
            n473 = call "BP Initialize.vi"("FP baud rate"=w852, "error in (no error)"=w868, "FrontPanel port"=w867) -> ("error out"=w866:errorcluster, "FrontPanel port"=w865:refnum<visa-resource-name>)  [unwired: 4 in]
            n474 = call "BP Get ID.vi"("error in (no error)"=w866, "FrontPanel port"=w865) -> ("error out"=w854:errorcluster, "Device ID string"=w858:string, "FrontPanel port"=w859:refnum<visa-resource-name>)  [unwired: 6 in, 1 out]
            n475 = local write "Panel ID"(w858) -> ()
            n476 = call "Get GHS version and type.vi"("ID string"=w858, "error in (no error)"=w854) -> ("Panel Version"=w861:bool, "System Type"=w863:bool, "error out"=w853:errorcluster)  [unwired: 4 in]
            n477 = Boolean To (0,1)(Boolean=w861) -> (0, 1=w862:i16)
            n478 = Boolean To (0,1)(Boolean=w863) -> (0, 1=w864:i16)
            n479 = property on="FP Layout" class="TabCtl (strict)"("Value"=w862) -> ()  [unwired: 2 in, 2 out]
            n480 = property on="Type" class="RadioBtnsControl (strict)"("Val(Sgnl)"=w864) -> ()  [unwired: 2 in, 2 out]
            n481 = call <userlib>:"Wait (ms)__ogtk.vi"("error in (no error)"=w853, "Wait on Error (FALSE)"=TRUE, "milliseconds to wait"=u32 1000) -> ("error out"=w857:errorcluster)  [unwired: 7 in, 1 out]
          }
        }
        n482 = local write "FP error"(w816) -> ()
        n483 = property on="FP port" class="VISAName"("Value"=w814) -> ()  [unwired: 2 in, 2 out]
      }
      n484 = call "MGI Clear Error.vi"() -> ("Error Out"=w762:errorcluster)  [unwired: 7 in]
      n485 = while {
        tunnel: w769 -> [w922]
        tunnel: w768 -> [w921]
        tunnel: w767 -> [w912]
        tunnel: w765 -> [w918]
        shift-right: [w911] -> _
        shift-left: w762 -> [w917]
        stop <- w915 stop-if-true
        # "Pulse Tube 1"
        n486 = case shown="True" w912 {
          tunnel: [dbl[] [0.0, 0.0, 0.0, 0.0, 0.0, 0.0, 0.0, 0.0] w939] -> w923
          tunnel: w922 -> [_ w938]
          tunnel: w917 -> [w924 w937]
          tunnel: w921 -> [_ w936]
          tunnel: w918 -> [_ w931]
          tunnel: [w924 w930] -> w910
          frame False {
          }
          frame True {
            n487 = call "PT Read Status.vi"("error in (no error)"=w937, "Baud"=w931, "Slave Address"=w936, "Com Port #"=w938) -> ("error out"=w930:errorcluster, "Response"=w940:T30)
            n488 = call "PT Parse Response.vi"("Response"=w940) -> ("Oil temp"=w945:T31, "He temp"=w944:cluster{"[2]":dbl, "[2]":dbl, "[2]":dbl, dbl}, "Out water temp"=w943:T32, "In water temp"=w942:T33, "P_low"=→"P Low":T33, "Numeric"=w949:i32, "P_high"=→"P High":T33, "Average pressure"=w935:cluster{"Low":dbl, "High":dbl}, "Current"=w929:cluster{"Current":dbl, "Threshold":dbl}, "PT Error"=w941:i32)  [unwired: 1 in]
            "Oil" <- w945
            "Motor" <- w929
            "PT Status" <- w949
            "Water Out" <- w943
            "Water In" <- w942
            "Helium" <- w944
            "P_avg" <- w935
            n489 = property on="PT Error" class="DigNum (strict)"("Val(Sgnl)"=w941) -> ()  [unwired: 2 in, 2 out]
            n490 = Unbundle By Name(w942) -> ("Values[0]"=w932:dbl)
            n491 = Unbundle By Name(w943) -> ("[1]"=w948:dbl)
            n492 = Unbundle By Name(w944) -> ("[2]"=w947:dbl)
            n493 = Unbundle By Name(w945) -> ("[3]"=w946:dbl)
            n494 = Unbundle By Name(w935) -> ("Low"=w934:dbl, "High"=w933:dbl)
            n495 = Unbundle By Name(w929) -> ("Current"=w928:dbl)
            n496 = Not Equal To 0?(x=w949) -> (x != 0?=w950:bool)
            n497 = Boolean To (0,1)(Boolean=w950) -> (0, 1=w951:i16)
            n498 = Build Array(w951, w932, w948, w947, w946, w934, w933, w928) -> (w939:dbl[])
          }
        }
        "PT1 error" <- w910
        n499 = local read "Stop"() -> (w914:bool)
        n500 = property on="Averages" class="DigNum (strict)"() -> ("Value"=w920:i32)  [unwired: 2 in, 2 out]
        n501 = Not(x=w912) -> (.not. x?=w913:bool)
        n502 = call "Running average.vi"("Window Size"=w920, "New values"=w923) -> ("Filterred"=→"PT1 Data":dbl[])  [unwired: 2 in]
        n503 = call "MGI Clear Error.vi"("Error In"=w910) -> ("Error Out"=w911:errorcluster)  [unwired: 6 in]
        n504 = Or(x=w914, y=w913) -> (x .or. y?=w915:bool)
        n505 = Wait (ms)(milliseconds to wait=u32 250) -> ()  [unwired: 1 out]
      }
      n506 = property on="PT2 Enabled?" class="Bool (strict)"() -> ("Value"=w755:bool)  [unwired: 2 in, 2 out]
      n507 = property on="PT2 Bauds" class="DigNum (strict)"() -> ("Value"=w754:u32)  [unwired: 2 in, 2 out]
      n508 = property on="PT2 Address" class="DigNum (strict)"() -> ("Value"=w756:u8)  [unwired: 2 in, 2 out]
      n509 = property on="PT2 port" class="VISAName"() -> ("Value"=w759:refnum<visa-resource-name>)  [unwired: 2 in, 2 out]
      n510 = call "VISA to RS232 Port Nr.vi"("VISA Resource Name"=w759) -> ("Port Number"=w758:u8)  [unwired: 1 in]
      n511 = Increment(x=w758) -> (x+1=w757:u8)
      n512 = call "MGI Clear Error.vi"() -> ("Error Out"=w753:errorcluster)  [unwired: 7 in]
      n513 = local read "MG error"() -> (w760:errorcluster)
      n514 = property on="Enabled?" class="Bool (strict)"() -> ("Value"=w766:bool)  [unwired: 2 in, 2 out]
      n515 = property on="MG port" class="VISAName"() -> ("Value"=w764:refnum<visa-resource-name>)  [unwired: 2 in, 2 out]
      n516 = while {
        tunnel: w757 -> [w784]
        tunnel: w756 -> [w783]
        tunnel: w755 -> [w774]
        tunnel: w754 -> [w780]
        shift-right: [w773] -> _
        shift-left: w753 -> [w779]
        stop <- w777 stop-if-true
        # "Pulse Tube 2"
        n517 = case shown="True" w774 {
          tunnel: [dbl[] [0.0, 0.0, 0.0, 0.0, 0.0, 0.0, 0.0, 0.0] w801] -> w785
          tunnel: w784 -> [_ w800]
          tunnel: w779 -> [w786 w799]
          tunnel: w783 -> [_ w798]
          tunnel: w780 -> [_ w793]
          tunnel: [w786 w792] -> w772
          frame False {
          }
          frame True {
            n518 = call "PT Read Status.vi"("error in (no error)"=w799, "Baud"=w793, "Slave Address"=w798, "Com Port #"=w800) -> ("error out"=w792:errorcluster, "Response"=w802:T30)
            n519 = call "PT Parse Response.vi"("Response"=w802) -> ("Oil temp"=w807:T31, "He temp"=w806:cluster{"[2]":dbl, "[2]":dbl, "[2]":dbl, dbl}, "Out water temp"=w805:T32, "In water temp"=w804:T33, "P_low"=→"P Low":T33, "Numeric"=w811:i32, "P_high"=→"P High":T33, "Average pressure"=w797:cluster{"Low":dbl, "High":dbl}, "Current"=w791:cluster{"Current":dbl, "Threshold":dbl}, "PT Error"=w803:i32)  [unwired: 1 in]
            "Oil" <- w807
            "Motor" <- w791
            "PT Status" <- w811
            "Water Out" <- w805
            "Water In" <- w804
            "Helium" <- w806
            "P_avg 2" <- w797
            n520 = property on="PT Error" class="DigNum (strict)"("Val(Sgnl)"=w803) -> ()  [unwired: 2 in, 2 out]
            n521 = Unbundle By Name(w804) -> ("Values[0]"=w794:dbl)
            n522 = Unbundle By Name(w805) -> ("[1]"=w810:dbl)
            n523 = Unbundle By Name(w806) -> ("[2]"=w809:dbl)
            n524 = Unbundle By Name(w807) -> ("[3]"=w808:dbl)
            n525 = Unbundle By Name(w797) -> ("Low"=w796:dbl, "High"=w795:dbl)
            n526 = Unbundle By Name(w791) -> ("Current"=w790:dbl)
            n527 = Not Equal To 0?(x=w811) -> (x != 0?=w812:bool)
            n528 = Boolean To (0,1)(Boolean=w812) -> (0, 1=w813:i16)
            n529 = Build Array(w813, w794, w810, w809, w808, w796, w795, w790) -> (w801:dbl[])
          }
        }
        "PT2 error" <- w772
        n530 = local read "Stop"() -> (w776:bool)
        n531 = property on="Averages" class="DigNum (strict)"() -> ("Value"=w782:i32)  [unwired: 2 in, 2 out]
        n532 = Not(x=w774) -> (.not. x?=w775:bool)
        n533 = call "Running average.vi"("Window Size"=w782, "New values"=w785) -> ("Filterred"=→"PT2 Data":dbl[])  [unwired: 2 in]
        n534 = call "MGI Clear Error.vi"("Error In"=w772) -> ("Error Out"=w773:errorcluster)  [unwired: 6 in]
        n535 = Or(x=w776, y=w775) -> (x .or. y?=w777:bool)
        n536 = Wait (ms)(milliseconds to wait=u32 250) -> ()  [unwired: 1 out]
      }
      n537 = while {
        tunnel: w766 -> [w871]
        shift-right: [w875] -> _
        shift-left: w760 -> [w874]
        shift-right: [w873] -> _
        shift-left: w764 -> [w876]
        stop <- w872 stop-if-true
        # "MaxiGauge"
        n538 = case shown="True" w871 {
          tunnel: w876 -> [w880 w884]
          tunnel: [w879 w883] -> w875
          tunnel: w874 -> [w879 w882]
          tunnel: [w880 w881] -> w873
          frame False {
          }
          frame True {
            n539 = case shown="No Error" w882 {
              selector: w882 -> [w891 _]
              tunnel: w884 -> [w899 w909]
              tunnel: [w885 w900] -> w883
              tunnel: [w898 w908] -> w881
              frame No Error {
                n540 = call "MG collect pressureinfo.vi"("error in"=w891, "MaxiGauge port"=w899) -> ("error out"=w896:T34, "sensor values"=w894:dbl[], "MaxiGauge port"=w890:refnum<visa-resource-name>, "sensor status info"=w889:string[])  [unwired: 4 in, 2 out]
                n541 = call "MG get errorstatus.vi"("error in"=w896, "MaxiGauge port"=w890) -> ("error out"=w886:T34, "MaxiGauge port"=w898:refnum<visa-resource-name>)  [unwired: 2 in, 2 out]
                n542 = property on="Averages" class="DigNum (strict)"() -> ("Value"=w893:i32)  [unwired: 2 in, 2 out]
                n543 = call "Running average.vi"("Window Size"=w893, "New values"=w894) -> ("Filterred"=w892:dbl[])  [unwired: 2 in]
                "MG Data" <- w892
                n544 = Array To Cluster(array=w889) -> (cluster=→"Sensors Status":T35)
                n545 = Array To Cluster(array=w892) -> (cluster=→"MG pressures":T36)
                n546 = call <userlib>:"Wait (ms)__ogtk.vi"("error in (no error)"=w886, "Wait on Error (FALSE)"=TRUE, "milliseconds to wait"=u32 500) -> ("error out"=w885:errorcluster)  [unwired: 7 in, 1 out]
              }
              frame Error {
                w904 = TRUE ("ID query")
                n547 = VISA Close(VISA resource name=w909) -> (error out=w907:errorcluster)  [unwired: 1 in]
                n548 = call "VISA Check port.vi"("error in (no error)"=w907, "VISA Resource Name in"=w909) -> ("error out"=w906:errorcluster, "VISA Resource Name out"=w905:refnum<visa-resource-name>)  [unwired: 8 in]
                n549 = call "MG initialize.vi"("error in (no error)"=w906, "MG query errorstatus"=w904, "ID query"=w904, "MaxiGauge port"=w905) -> ("error out"=w901:errorcluster, "MaxiGauge port"=w908:refnum<visa-resource-name>)  [unwired: 2 in, 1 out]
                n550 = call <userlib>:"Wait (ms)__ogtk.vi"("error in (no error)"=w901, "Wait on Error (FALSE)"=TRUE, "milliseconds to wait"=u32 1000) -> ("error out"=w900:errorcluster)  [unwired: 7 in, 1 out]
              }
            }
          }
        }
        n551 = local read "Stop"() -> (w877:bool)
        n552 = Not(x=w871) -> (.not. x?=w870:bool)
        n553 = Or(x=w870, y=w877) -> (x .or. y?=w872:bool)
        n554 = local write "MG error"(w875) -> ()
        n555 = property on="MG port" class="VISAName"("Value"=w873) -> ()  [unwired: 2 in, 2 out]
        n556 = Wait (ms)(milliseconds to wait=u32 500) -> ()  [unwired: 1 out]
      }
    }
    frame #2 {
      n557 = Set Occurrence(w952) -> ()
    }
  }
